vi "BRig_RT__Case_Exp__State_initTrial__v18.vi"(0 "input_dataCurrent":u16[](array[numeric]), 9 "input_dataBlock":u16[][](array[numeric]), 11 "input_dataTrial":u16[][](array[numeric]), 12 "input_dataExp":u16[](array[numeric])) -> (1 "output_iTrial":u16, 2 "output_nTrial":u16, 3 "output_SolenoidReward":bool, 4 "output_dataCurrent":u16[](array[numeric]), 10 "output_dataBlock":u16[][](array[numeric]), 15 "output_dataTrial":u16[][](array[numeric]))   [LabVIEW 2014]
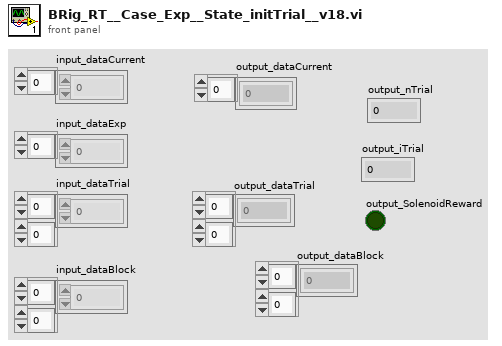
[diagram p1: front panel]
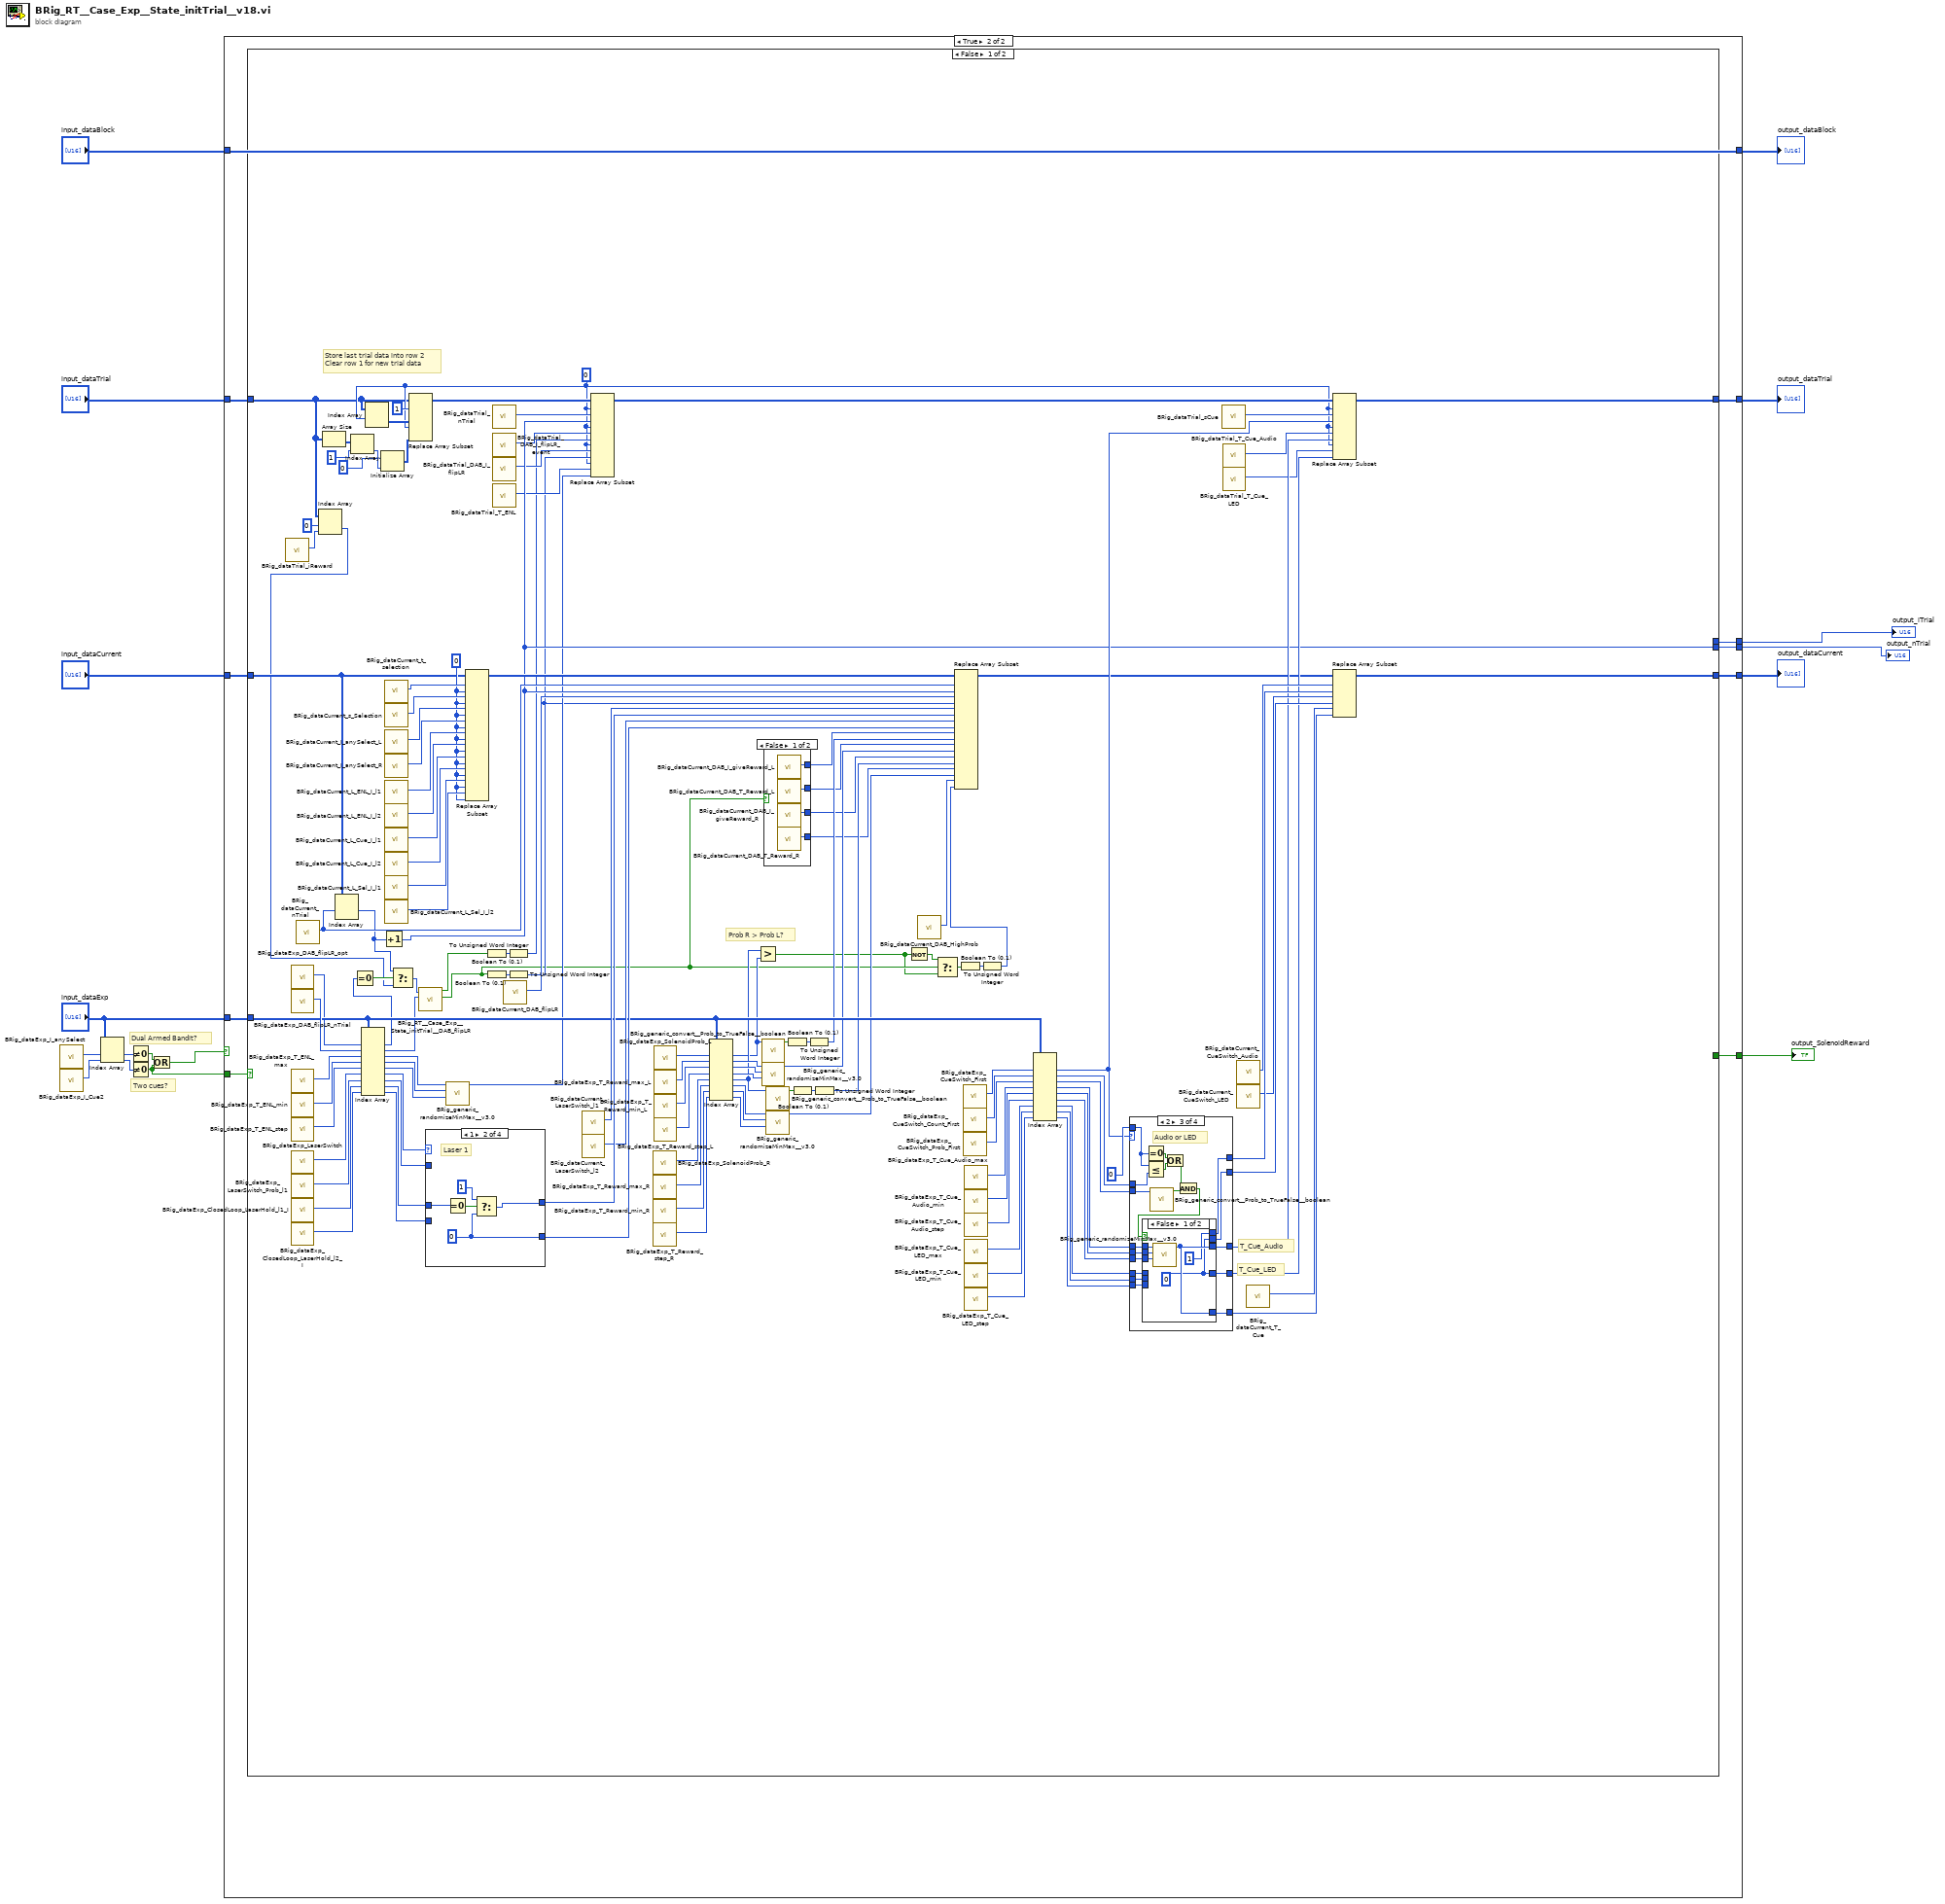
[diagram p0: block diagram]
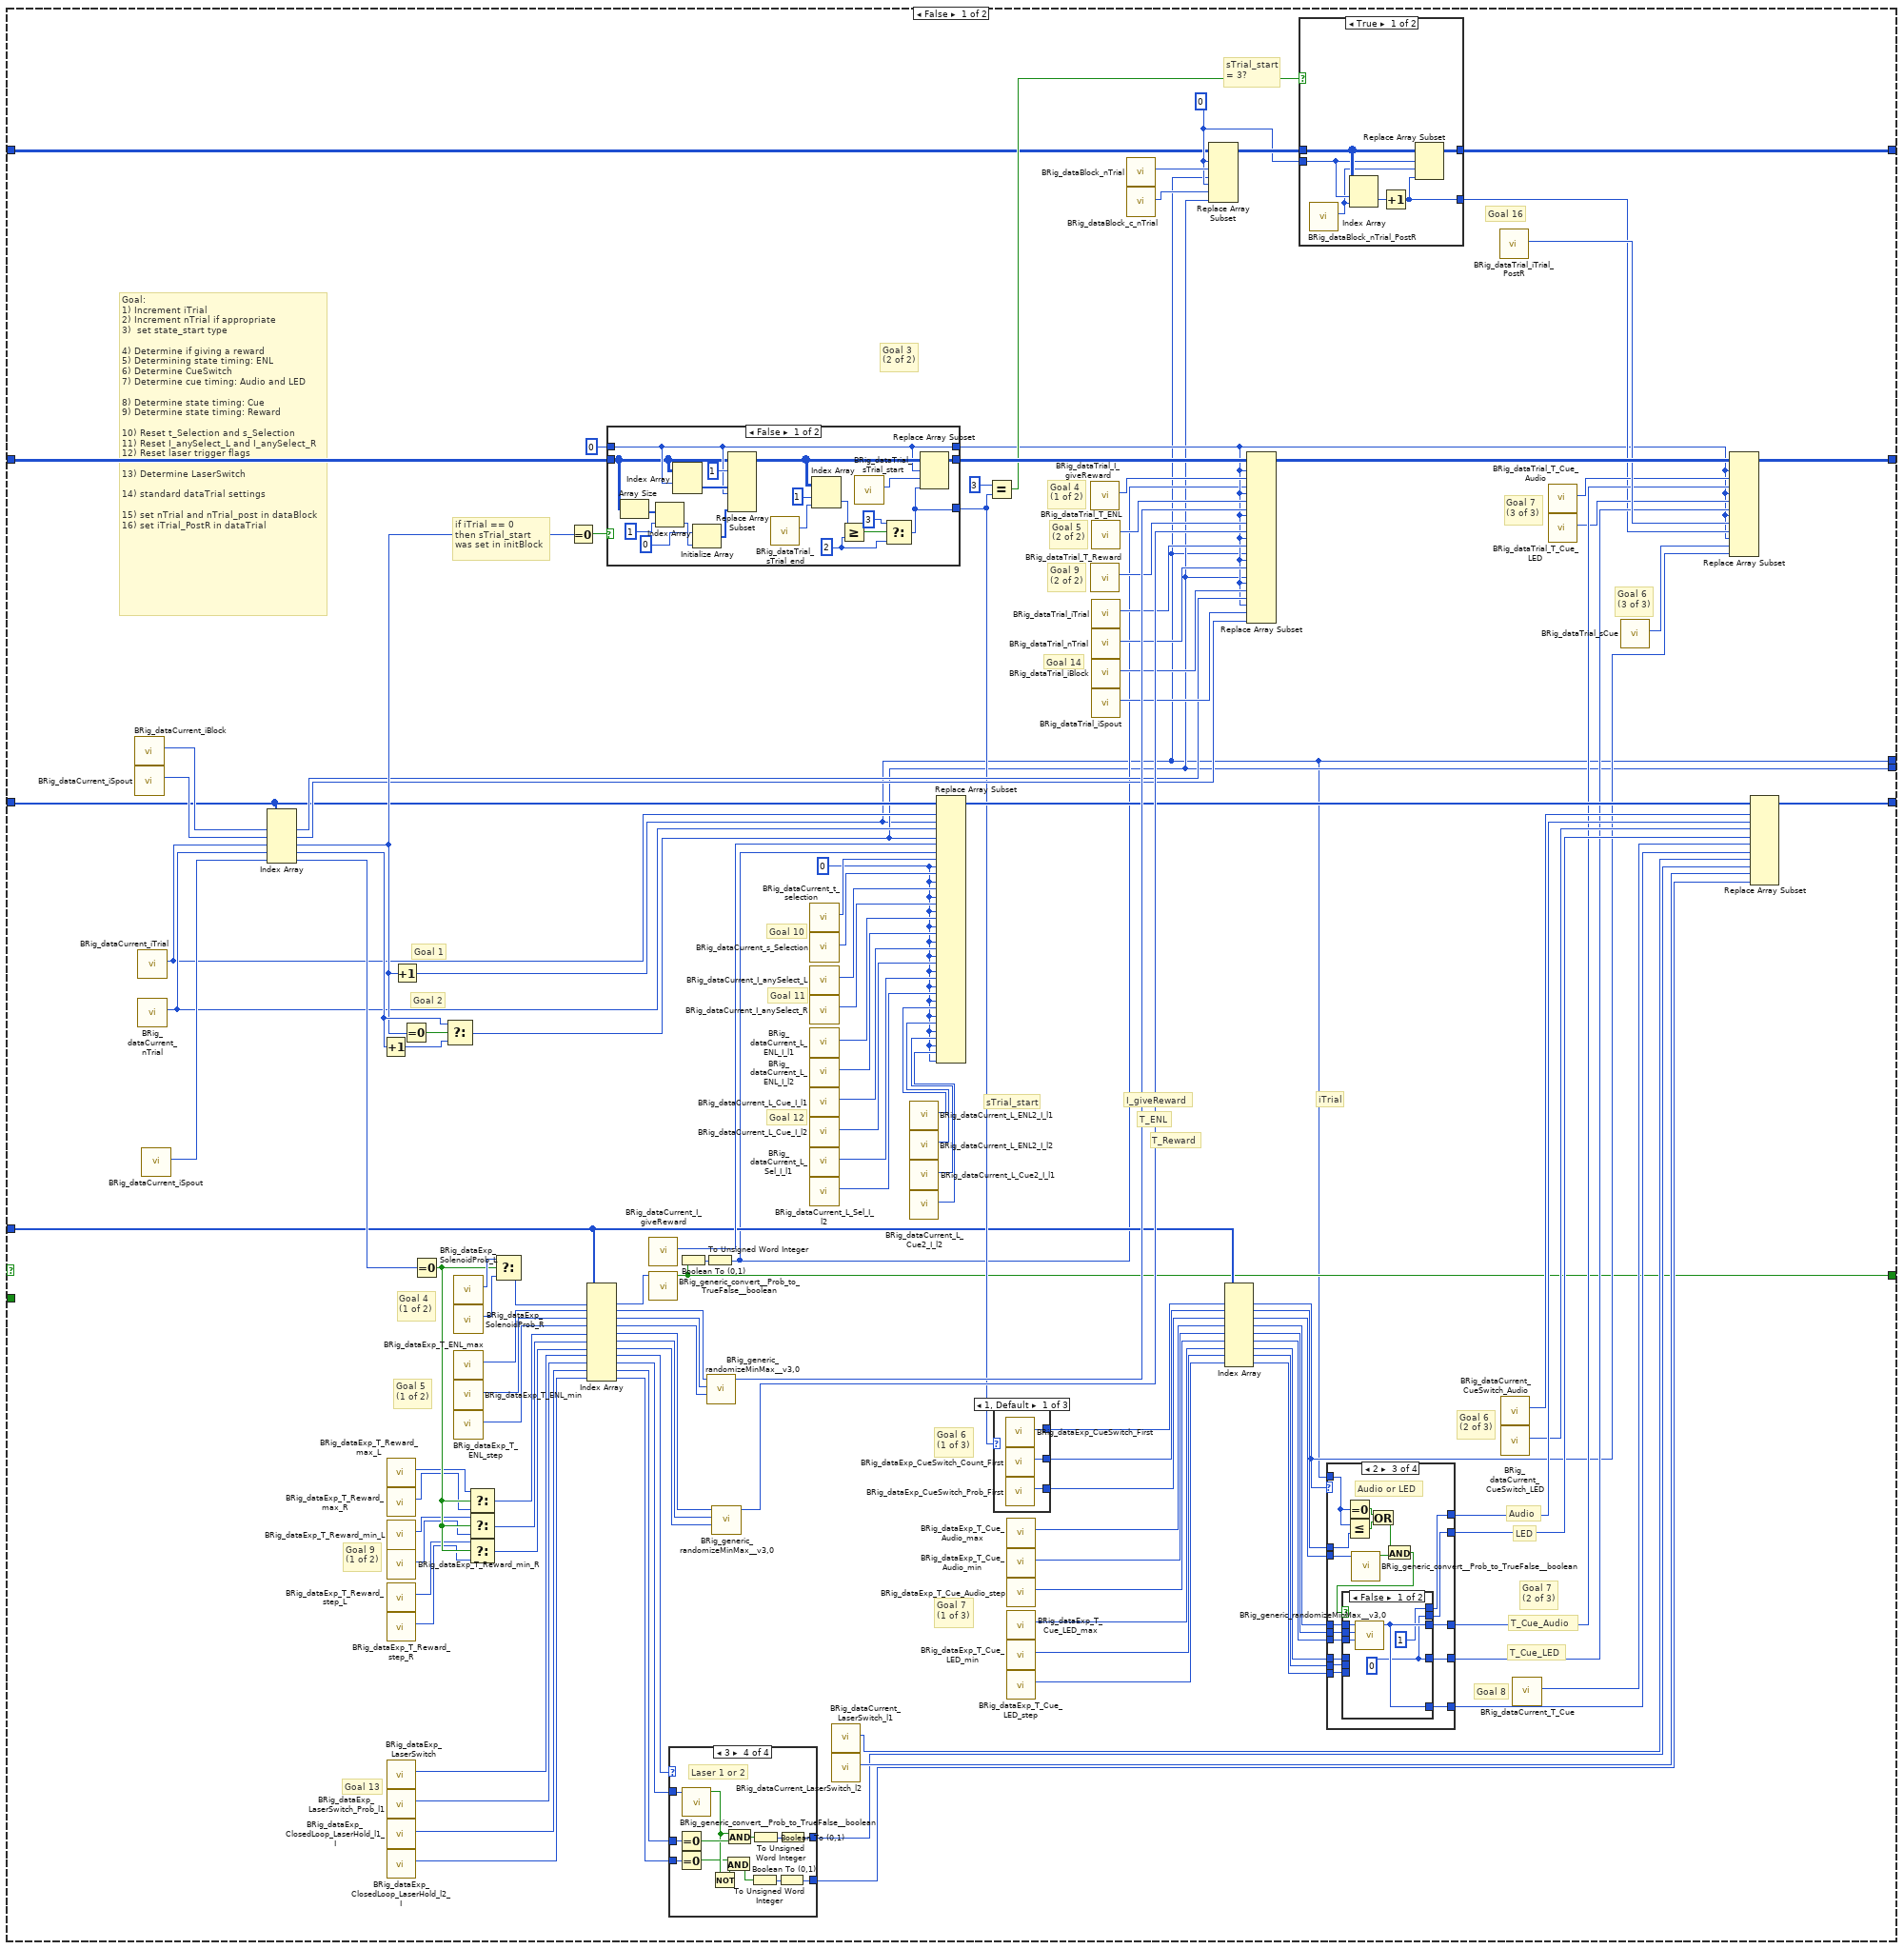
[diagram p2: hidden frame]
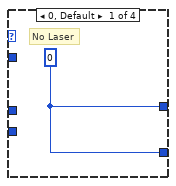
[diagram p4: hidden frame]
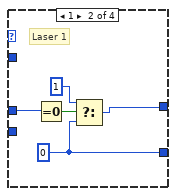
[diagram p5: hidden frame]
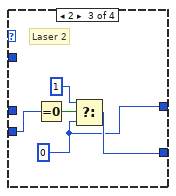
[diagram p6: hidden frame]
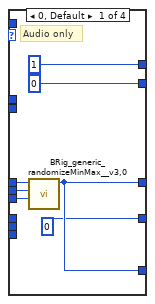
[diagram p7: hidden frame]
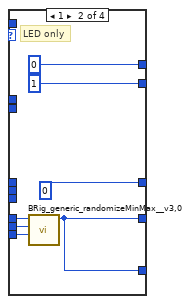
[diagram p8: hidden frame]
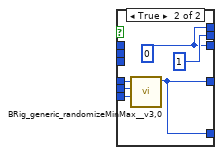
[diagram p9: hidden frame]
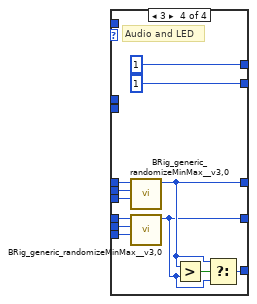
[diagram p10: hidden frame]
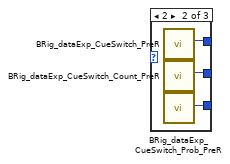
[diagram p11: hidden frame]
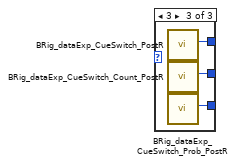
[diagram p12: hidden frame]
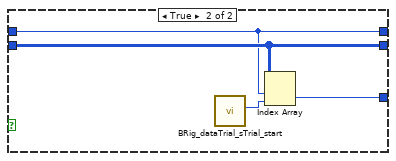
[diagram p13: hidden frame]
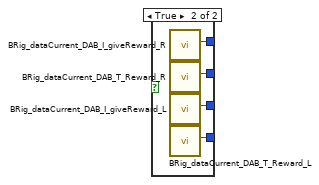
[diagram p14: hidden frame]
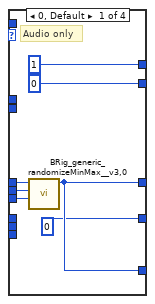
[diagram p15: hidden frame]
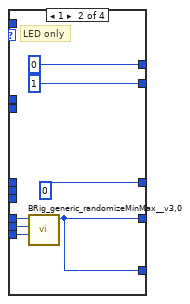
[diagram p16: hidden frame]
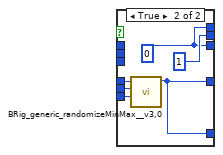
[diagram p17: hidden frame]
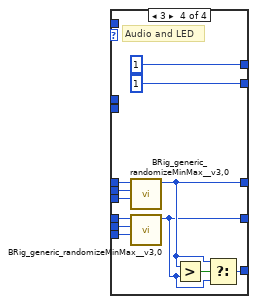
[diagram p18: hidden frame]
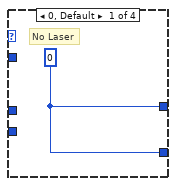
[diagram p19: hidden frame]
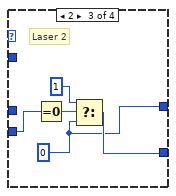
[diagram p20: hidden frame]
diagram:
  # "Two cues?"
  # "Dual Armed Bandit?"
  n1 = call "BRig_dataExp_I_anySelect.vi"() -> ("output_I_anySelect"=w8:i32)  [unwired: 11 in]
  n2 = call "BRig_dataExp_I_Cue2.vi"() -> ("output_I_Cue2"=w6:i32)  [unwired: 11 in]
  n3 = Index Array(array="input_dataExp", index #1=w8, index #2=w6) -> (element #1=w7:u16, element #2=w5:u16)
  n4 = Not Equal To 0?(x=w7) -> (x != 0?=w4:bool)
  n5 = Not Equal To 0?(x=w5) -> (x != 0?=w1:bool)
  n6 = Or(x=w4, y=w1) -> (x .or. y?=w2:bool)
  n7 = case shown="True" w2 {
    tunnel: "input_dataExp" -> [w28 w271]
    tunnel: "input_dataCurrent" -> [w27 w272]
    tunnel: "input_dataTrial" -> [w26 w269]
    tunnel: "input_dataBlock" -> [w25 w275]
    tunnel: [w24 w275] -> w14
    tunnel: [w23 w273] -> w13
    tunnel: [w22 w274] -> w12
    tunnel: [w21 w267] -> w11
    tunnel: [w19 w270] -> w10
    tunnel: [w18 w266] -> w9
    tunnel: w1 -> [_ w268]
    frame False {
      w39 = 0 ("disabled index (row)")
      w31 = u16 0 ("new element/subarray")
      # "Goal 16"
      # "Goal 6\n(3 of 3)"
      # "sTrial_start\n= 3?"
      # "Goal 14"
      # "Goal 13"
      # "iTrial"
      # "Goal 8"
      # "Goal 7\n(3 of 3)"
      # "Goal 7\n(2 of 3)"
      # "Goal 7\n(1 of 3)"
      # "T_Cue_LED"
      # "T_Cue_Audio"
      # "I_giveReward"
      # "Goal 4\n(1 of 2)"
      # "T_Reward"
      # "Goal 9\n(2 of 2)"
      # "Goal 9\n(1 of 2)"
      # "Goal 12"
      # "Goal 11"
      # "Goal 10"
      # "T_ENL"
      # "sTrial_start"
      # "LED"
      # "Audio"
      # "Goal 6\n(2 of 3)"
      # "Goal 6\n(1 of 3)"
      # "Goal 3\n(2 of 2)"
      # "Goal 5\n(2 of 2)"
      # "Goal 5\n(1 of 2)"
      # "Goal 4\n(1 of 2)"
      # "if iTrial == 0\nthen sTrial_start\nwas set in initBlock"
      # "Goal 2"
      # "Goal 1"
      # "Goal:\n1) Increment iTrial\n2) Increment nTrial if appropriate\n3)  set state_start type\n\n4) Determine if giving a reward\n5) Determining state timing: ENL\n6) Determine CueSwitch\n7) Determine cue timing: Audio and LED\n\n8) Determine state timing: Cue\n9) Determine state timing: Reward\n\n10) Reset t_Selection and s_Selection\n11) Reset I_anySelect_L and I_anySelect_R\n12) Reset laser trigger flags\n\n13) Determine LaserSwitch\n\n14) standard dataTrial settings\n\n15) set nTrial and nTrial_post in dataBlock\n16) set iTrial_PostR in dataTrial"
      n8 = call "BRig_dataCurrent_iBlock.vi"() -> ("output_iBlock"=w55:i32)  [unwired: 11 in]
      n9 = call "BRig_dataCurrent_iSpout.vi"() -> ("output_iSpout"=w54:i32)  [unwired: 11 in]
      n10 = call "BRig_dataCurrent_iTrial.vi"() -> ("output_iTrial"=w36:i32)  [unwired: 11 in]
      n11 = call "BRig_dataCurrent_nTrial.vi"() -> ("output_nTrial"=w37:i32)  [unwired: 11 in]
      n12 = call "BRig_dataCurrent_iSpout.vi"() -> ("output_iSpout"=w46:i32)  [unwired: 11 in]
      n13 = Index Array(array=w27, index #1=w55, index #2=w54, index #3=w36, index #4=w37, index #5=w46) -> (element #1=w64:u16, element #2=w63:u16, element #3=w77:u16, element #4=w144:u16, element #5=w45:u16)
      n14 = Increment(x=w144) -> (x+1=w143:u16)
      n15 = call "BRig_dataExp_T_Reward_max_L.vi"() -> ("output_T_Reward_max_L"=w108:i32)  [unwired: 11 in]
      n16 = call "BRig_dataExp_T_Reward_max_R.vi"() -> ("output_T_Reward_max_R"=w107:i32)  [unwired: 11 in]
      n17 = call "BRig_dataExp_T_Reward_min_L.vi"() -> ("output_Tcycle_Reward_min_L"=w106:i32)  [unwired: 11 in]
      n18 = call "BRig_dataExp_T_Reward_min_R.vi"() -> ("output_T_Reward_min_R"=w105:i32)  [unwired: 11 in]
      n19 = call "BRig_dataExp_T_Reward_step_L.vi"() -> ("output_T_Reward_step_L"=w104:i32)  [unwired: 11 in]
      n20 = call "BRig_dataExp_T_Reward_step_R.vi"() -> ("output_T_Reward_step_R"=w103:i32)  [unwired: 11 in]
      n21 = call "BRig_dataExp_LaserSwitch.vi"() -> ("output_LaserSwitch"=w76:i32)  [unwired: 11 in]
      n22 = call "BRig_dataExp_LaserSwitch_Prob_l1.vi"() -> ("output_LaserSwitch_Probability_L1"=w75:i32)  [unwired: 11 in]
      n23 = call "BRig_dataExp_ClosedLoop_LaserHold_l1_I.vi"() -> ("output_CloseLoop_LaserHold_l1_I"=w51:i32)  [unwired: 11 in]
      n24 = call "BRig_dataExp_ClosedLoop_LaserHold_l2_I.vi"() -> ("output_CloseLoop_LaserHold_l2_I"=w50:i32)  [unwired: 11 in]
      n25 = Increment(x=w77) -> (x+1=w18:u16)
      n26 = Equal To 0?(x=w77) -> (x = 0?=w142:bool)
      n27 = Equal To 0?(x=w45) -> (x = 0?=w109:bool)
      n28 = Select(t=w144, s=w142, f=w143) -> (s? t:f=w19:u16)
      n29 = call "BRig_dataExp_SolenoidProb_L.vi"() -> ("output_SolenoidProbability_L"=w139:i32)  [unwired: 11 in]
      n30 = call "BRig_dataExp_SolenoidProb_R.vi"() -> ("output_SolenoidProbability_R"=w138:i32)  [unwired: 11 in]
      n31 = call "BRig_dataExp_T_ENL_max.vi"() -> ("output_T_ENL_max"=w133:i32)  [unwired: 11 in]
      n32 = call "BRig_dataExp_T_ENL_min.vi"() -> ("output_T_ENL_min"=w134:i32)  [unwired: 11 in]
      n33 = call "BRig_dataExp_T_ENL_step.vi"() -> ("output_T_ENL_step"=w135:i32)  [unwired: 11 in]
      n34 = Select(t=w108, s=w109, f=w107) -> (s? t:f=w102:i32)
      n35 = Select(t=w106, s=w109, f=w105) -> (s? t:f=w101:i32)
      n36 = Select(t=w104, s=w109, f=w103) -> (s? t:f=w100:i32)
      n37 = Select(t=w139, s=w109, f=w138) -> (s? t:f=w137:i32)
      n38 = Equal To 0?(x=w77) -> (x = 0?=w141:bool)
      n39 = Index Array(array=w28, index #1=w137, index #2=w133, index #3=w134, index #4=w135, index #5=w102, index #6=w101, index #7=w100, index #8=w76, index #9=w75, index #10=w51, index #11=w50) -> (element #1=w136:u16, element #2=w132:u16, element #3=w131:u16, element #4=w130:u16, element #5=w99:u16, element #6=w98:u16, element #7=w97:u16, element #8=w74:u16, element #9=w73:u16, element #10=w49:u16, element #11=w48:u16)
      n40 = case shown="False" w141 {
        tunnel: w26 -> [w248 w265]
        tunnel: [w259 w265] -> w129
        tunnel: 0 -> [w249 w264]
        tunnel: [w249 w264] -> w29
        tunnel: [w255 w262] -> w30
        frame False {
          w256 = u16 2 ("y")
          n41 = Array Size(array=w248) -> (size(s)=w247:i32[])
          n42 = Index Array(array=w247, index=1) -> (element=w245:i32)
          n43 = Index Array(array=w248, index (row)=w249) -> (element=w252:u16[])  [unwired: 1 in]
          n44 = Initialize Array(u16 0 ("index"), w245) -> (w243:u16[])
          n45 = Replace Array Subset(array=w248, new element #1=w252, index (row) #1=1 ("index (row)"), new element #2=w243, index (row) #2=w249) -> (w250:u16[][])  [unwired: 2 in]
          n46 = call "BRig_dataTrial_sTrial_end.vi"() -> ("output_sTrial_end"=w261:i32)  [unwired: 11 in]
          n47 = Index Array(array=w250, index (row)=1 ("disabled index (row)"), index (col)=w261) -> (element=w260:u16)
          n48 = Greater Or Equal?(x=w260, y=w256) -> (x >= y?=w258:bool)
          n49 = call "BRig_dataTrial_sTrial_start.vi"() -> ("output_sTrial_start"=w254:i32)  [unwired: 11 in]
          n50 = Select(t=u16 3 ("y"), s=w258, f=w256) -> (s? t:f=w255:u16)
          n51 = Replace Array Subset(array=w250, new element=w255, index (row)=w249, index (col)=w254) -> (w259:u16[][])
        }
        frame True {
          n52 = call "BRig_dataTrial_sTrial_start.vi"() -> ("output_sTrial_start"=w263:i32)  [unwired: 11 in]
          n53 = Index Array(array=w265, index (row)=w264, index (col)=w263) -> (element=w262:u16)
        }
      }
      n54 = call "BRig_dataCurrent_I_giveReward.vi"() -> ("output_I_giveReward"=w140:i32)  [unwired: 11 in]
      n55 = call "BRig_generic_convert__Prob_to_TrueFalse__boolean.vi"("input_probability_u16"=w136) -> ("output_TF"=w21:bool)  [unwired: 10 in]
      n56 = case shown="3" w74 {
        tunnel: [w153 w154 w159 w173] -> w71
        tunnel: [w153 w155 w160 w172] -> w70
        tunnel: w73 -> [_ _ _ w176]
        tunnel: w49 -> [_ w158 _ w171]
        tunnel: w48 -> [_ _ w161 w170]
        frame 0, Default {
          w153 = u16 0
          # "No Laser"
        }
        frame 1 {
          w155 = u16 0
          # "Laser 1"
          n57 = Equal To 0?(x=w158) -> (x = 0?=w157:bool)
          n58 = Select(t=u16 1, s=w157, f=w155) -> (s? t:f=w154:u16)
        }
        frame 2 {
          w159 = u16 0
          # "Laser 2"
          n59 = Equal To 0?(x=w161) -> (x = 0?=w163:bool)
          n60 = Select(t=u16 1, s=w163, f=w159) -> (s? t:f=w160:u16)
        }
        frame 3 {
          # "Laser 1 or 2"
          n61 = Equal To 0?(x=w171) -> (x = 0?=w169:bool)
          n62 = Equal To 0?(x=w170) -> (x = 0?=w165:bool)
          n63 = call "BRig_generic_convert__Prob_to_TrueFalse__boolean.vi"("input_probability_u16"=w176) -> ("output_TF"=w168:bool)  [unwired: 10 in]
          n64 = Not(x=w168) -> (.not. x?=w166:bool)
          n65 = And(x=w165, y=w166) -> (x .and. y?=w164:bool)
          n66 = And(x=w168, y=w169) -> (x .and. y?=w167:bool)
          n67 = Boolean To (0,1)(Boolean=w164) -> (0, 1=w175:i16)
          n68 = Boolean To (0,1)(Boolean=w167) -> (0, 1=w174:i16)
          n69 = To Unsigned Word Integer(number=w175) -> (unsigned 16bit integer=w172:u16)
          n70 = To Unsigned Word Integer(number=w174) -> (unsigned 16bit integer=w173:u16)
        }
      }
      n71 = Boolean To (0,1)(Boolean=w21) -> (0, 1=w145:i16)
      n72 = To Unsigned Word Integer(number=w145) -> (unsigned 16bit integer=w20:u16)
      n73 = call "BRig_generic_randomizeMinMax__v3,0.vi"("Input_Increment"=w130, "Input_Min"=w131, "Input_Max"=w132) -> ("Output"=w127:u16)  [unwired: 8 in]
      n74 = call "BRig_generic_randomizeMinMax__v3,0.vi"("Input_Increment"=w97, "Input_Min"=w98, "Input_Max"=w99) -> ("Output"=w95:u16)  [unwired: 8 in]
      n75 = call "BRig_dataCurrent_t_selection.vi"() -> ("output_t_selection"=w119:i32)  [unwired: 11 in]
      n76 = call "BRig_dataCurrent_s_Selection.vi"() -> ("output_s_Selection"=w118:i32)  [unwired: 11 in]
      n77 = call "BRig_dataCurrent_I_anySelect_L.vi"() -> ("output_IanySelect_L"=w117:i32)  [unwired: 11 in]
      n78 = call "BRig_dataCurrent_I_anySelect_R.vi"() -> ("output_IanySelect_R"=w116:i32)  [unwired: 11 in]
      n79 = call "BRig_dataCurrent_L_ENL_I_l1.vi"() -> ("output_L_ENL_I_l1"=w115:i32)  [unwired: 11 in]
      n80 = call "BRig_dataCurrent_L_ENL_I_l2.vi"() -> ("output_L_ENL_I_l2"=w114:i32)  [unwired: 11 in]
      n81 = call "BRig_dataCurrent_L_Cue_I_l1.vi"() -> ("output_L_Cue_I_l1"=w113:i32)  [unwired: 11 in]
      n82 = call "BRig_dataCurrent_L_Cue_I_l2.vi"() -> ("output_L_Cue_I_l2"=w112:i32)  [unwired: 11 in]
      n83 = call "BRig_dataCurrent_L_Sel_I_l1.vi"() -> ("output_L_Sel_I_l1"=w111:i32)  [unwired: 11 in]
      n84 = call "BRig_dataCurrent_L_Sel_I_l2.vi"() -> ("output_L_Sel_I_l2"=w110:i32)  [unwired: 11 in]
      n85 = call "BRig_dataCurrent_LaserSwitch_l1.vi"() -> ("output_LaserSwitch_l1"=w69:i32)  [unwired: 11 in]
      n86 = call "BRig_dataCurrent_LaserSwitch_l2.vi"() -> ("output_LaserSwitch_l2"=w72:i32)  [unwired: 11 in]
      n87 = call "BRig_dataCurrent_L_ENL2_I_l1.vi"() -> ("output_L_ENL2_I_l1"=w35:i32)  [unwired: 11 in]
      n88 = call "BRig_dataCurrent_L_ENL2_I_l2.vi"() -> ("output_L_ENL2_I_l2"=w34:i32)  [unwired: 11 in]
      n89 = call "BRig_dataCurrent_L_Cue2_I_l1.vi"() -> ("output_L_Cue2_I_l1"=w33:i32)  [unwired: 11 in]
      n90 = call "BRig_dataCurrent_L_Cue2_I_l2.vi"() -> ("output_L_Cue2_I_l2"=w32:i32)  [unwired: 11 in]
      n91 = Replace Array Subset(array=w27, new element #1=w18, index #1=w36, new element #2=w19, index #2=w37, new element #3=w20, index #3=w140, new element #4=w31, index #4=w119, new element #5=w31, index #5=w118, new element #6=w31, index #6=w117, new element #7=w31, index #7=w116, new element #8=w31, index #8=w115, new element #9=w31, index #9=w114, new element #10=w31, index #10=w113, new element #11=w31, index #11=w112, new element #12=w31, index #12=w111, new element #13=w31, index #13=w110, new element #14=w31, index #14=w35, new element #15=w31, index #15=w34, new element #16=w31, index #16=w33, new element #17=w31, index #17=w32) -> (w62:u16[])
      n92 = Equal?(x=u16 3 ("y"), y=w30) -> (x = y?=w40:bool)
      n93 = case shown="1, Default" w30 {
        tunnel: [w236 w237 w242] -> w126
        tunnel: [w235 w238 w241] -> w125
        tunnel: [w234 w239 w240] -> w124
        frame 1, Default {
          n94 = call "BRig_dataExp_CueSwitch_First.vi"() -> ("output_CueSwitch_First"=w236:i32)  [unwired: 11 in]
          n95 = call "BRig_dataExp_CueSwitch_Count_First.vi"() -> ("output_CueSwitch_Count_First"=w235:i32)  [unwired: 11 in]
          n96 = call "BRig_dataExp_CueSwitch_Prob_First.vi"() -> ("output_CueSwitch_Prob_First"=w234:i32)  [unwired: 11 in]
        }
        frame 2 {
          n97 = call "BRig_dataExp_CueSwitch_PreR.vi"() -> ("output_CueSwitch_PreR"=w237:i32)  [unwired: 11 in]
          n98 = call "BRig_dataExp_CueSwitch_Count_PreR.vi"() -> ("output_CueSwitch_Count_PreR"=w238:i32)  [unwired: 11 in]
          n99 = call "BRig_dataExp_CueSwitch_Prob_PreR.vi"() -> ("output_CueSwitch_Prob_PreR"=w239:i32)  [unwired: 11 in]
        }
        frame 3 {
          n100 = call "BRig_dataExp_CueSwitch_PostR.vi"() -> ("output_CueSwitch_PostR"=w242:i32)  [unwired: 11 in]
          n101 = call "BRig_dataExp_CueSwitch_Count_PostR.vi"() -> ("output_CueSwitch_Count_PostR"=w241:i32)  [unwired: 11 in]
          n102 = call "BRig_dataExp_CueSwitch_Prob_PostR.vi"() -> ("output_CueSwitch_Prob_PostR"=w240:i32)  [unwired: 11 in]
        }
      }
      n103 = call "BRig_dataExp_T_Cue_Audio_max.vi"() -> ("output_T_Cue_Audio_max"=w93:i32)  [unwired: 11 in]
      n104 = call "BRig_dataExp_T_Cue_Audio_min.vi"() -> ("output_T_Cue_Audio_min"=w92:i32)  [unwired: 11 in]
      n105 = call "BRig_dataExp_T_Cue_Audio_step.vi"() -> ("output_T_Cue_Audio_step"=w91:i32)  [unwired: 11 in]
      n106 = call "BRig_dataExp_T_Cue_LED_max.vi"() -> ("output_T_Cue_LED_max"=w90:i32)  [unwired: 11 in]
      n107 = call "BRig_dataExp_T_Cue_LED_min.vi"() -> ("output_T_Cue_LED_min"=w89:i32)  [unwired: 11 in]
      n108 = call "BRig_dataExp_T_Cue_LED_step.vi"() -> ("output_T_Cue_LED_step"=w88:i32)  [unwired: 11 in]
      n109 = call "BRig_dataTrial_I_giveReward.vi"() -> ("output_I_giveReward"=w94:i32)  [unwired: 11 in]
      n110 = call "BRig_dataTrial_T_Reward.vi"() -> ("output_T_Reward"=w96:i32)  [unwired: 11 in]
      n111 = call "BRig_dataTrial_T_ENL.vi"() -> ("output_T_ENL"=w128:i32)  [unwired: 11 in]
      n112 = call "BRig_dataTrial_iTrial.vi"() -> ("output_iTrial"=w68:i32)  [unwired: 11 in]
      n113 = call "BRig_dataTrial_nTrial.vi"() -> ("output_nTrial"=w67:i32)  [unwired: 11 in]
      n114 = call "BRig_dataTrial_iBlock.vi"() -> ("output_iBlock"=w66:i32)  [unwired: 11 in]
      n115 = call "BRig_dataTrial_iSpout.vi"() -> ("output_iSpout"=w65:i32)  [unwired: 11 in]
      n116 = call "BRig_dataBlock_nTrial.vi"() -> ("output_nTrial"=w42:i32)  [unwired: 11 in]
      n117 = call "BRig_dataBlock_c_nTrial.vi"() -> ("output_c_nTrial"=w41:i32)  [unwired: 11 in]
      n118 = Replace Array Subset(array=w25, new element #1=w18, index (row) #1=w39, index (col) #1=w42, new element #2=w19, index (row) #2=w39, index (col) #2=w41) -> (w43:u16[][])
      n119 = Index Array(array=w28, index #1=w126, index #2=w125, index #3=w124, index #4=w93, index #5=w92, index #6=w91, index #7=w90, index #8=w89, index #9=w88) -> (element #1=w52:u16, element #2=w87:u16, element #3=w86:u16, element #4=w85:u16, element #5=w84:u16, element #6=w83:u16, element #7=w82:u16, element #8=w81:u16, element #9=w80:u16)
      n120 = Replace Array Subset(array=w129, new element #1=w20, index (row) #1=w29, index (col) #1=w94, new element #2=w127, index (row) #2=w29, index (col) #2=w128, new element #3=w95, index (row) #3=w29, index (col) #3=w96, new element #4=w18, index (row) #4=w29, index (col) #4=w68, new element #5=w19, index (row) #5=w29, index (col) #5=w67, new element #6=w64, index (row) #6=w29, index (col) #6=w66, new element #7=w63, index (row) #7=w29, index (col) #7=w65) -> (w61:u16[][])
      n121 = case shown="True" w40 {
        tunnel: w43 -> [w151 w152]
        tunnel: [w149 w152] -> w24
        tunnel: [w146 _] -> w38
        tunnel: w39 -> [w148 _]
        frame True {
          n122 = call "BRig_dataBlock_nTrial_PostR.vi"() -> ("output_nTrial_PostR"=w147:i32)  [unwired: 11 in]
          n123 = Index Array(array=w151, index (row)=w148, index (col)=w147) -> (element=w150:u16)
          n124 = Increment(x=w150) -> (x+1=w146:u16)
          n125 = Replace Array Subset(array=w151, new element=w146, index (row)=w148, index (col)=w147) -> (w149:u16[][])
        }
        frame False {
        }
      }
      n126 = case shown="2" w52 {
        tunnel: [u16 1 u16 0 w195 u16 1] -> w122
        tunnel: [u16 0 u16 1 w194 u16 1] -> w120
        tunnel: w87 -> [_ _ w208 _]
        tunnel: w86 -> [_ _ w205 _]
        tunnel: w85 -> [w181 _ w201 w231]
        tunnel: w84 -> [w180 _ w200 w230]
        tunnel: w83 -> [w179 _ w199 w229]
        tunnel: w82 -> [_ w188 w193 w228]
        tunnel: w81 -> [_ w187 w192 w227]
        tunnel: w80 -> [_ w186 w191 w226]
        tunnel: [w178 u16 0 ("Output") w198 w224] -> w59
        tunnel: [u16 0 ("Output") w185 w196 w223] -> w58
        tunnel: [w178 w185 w197 w222] -> w78
        tunnel: w18 -> [_ _ w209 _]
        frame 0, Default {
          # "Audio only"
          n127 = call "BRig_generic_randomizeMinMax__v3,0.vi"("Input_Increment"=w179, "Input_Min"=w180, "Input_Max"=w181) -> ("Output"=w178:u16)  [unwired: 8 in]
        }
        frame 1 {
          # "LED only"
          n128 = call "BRig_generic_randomizeMinMax__v3,0.vi"("Input_Increment"=w186, "Input_Min"=w187, "Input_Max"=w188) -> ("Output"=w185:u16)  [unwired: 8 in]
        }
        frame 2 {
          # "Audio or LED"
          n129 = Equal To 0?(x=w209) -> (x = 0?=w207:bool)
          n130 = Less Or Equal?(x=w209, y=w208) -> (x <= y?=w206:bool)
          n131 = call "BRig_generic_convert__Prob_to_TrueFalse__boolean.vi"("input_probability_u16"=w205) -> ("output_TF"=w204:bool)  [unwired: 10 in]
          n132 = Or(x=w207, y=w206) -> (x .or. y?=w203:bool)
          n133 = And(x=w203, y=w204) -> (x .and. y?=w202:bool)
          n134 = case shown="False" w202 {
            tunnel: w201 -> [w215 _]
            tunnel: w200 -> [w214 _]
            tunnel: w199 -> [w213 _]
            tunnel: [w212 w216] -> w198
            tunnel: [w212 w218] -> w197
            tunnel: [w210 w218] -> w196
            tunnel: [u16 1 w216] -> w195
            tunnel: [w210 u16 1] -> w194
            tunnel: w193 -> [_ w221]
            tunnel: w192 -> [_ w220]
            tunnel: w191 -> [_ w219]
            frame False {
              w210 = u16 0
              n135 = call "BRig_generic_randomizeMinMax__v3,0.vi"("Input_Increment"=w213, "Input_Min"=w214, "Input_Max"=w215) -> ("Output"=w212:u16)  [unwired: 8 in]
            }
            frame True {
              w216 = u16 0
              n136 = call "BRig_generic_randomizeMinMax__v3,0.vi"("Input_Increment"=w219, "Input_Min"=w220, "Input_Max"=w221) -> ("Output"=w218:u16)  [unwired: 8 in]
            }
          }
        }
        frame 3 {
          # "Audio and LED"
          n137 = call "BRig_generic_randomizeMinMax__v3,0.vi"("Input_Increment"=w229, "Input_Min"=w230, "Input_Max"=w231) -> ("Output"=w224:u16)  [unwired: 8 in]
          n138 = call "BRig_generic_randomizeMinMax__v3,0.vi"("Input_Increment"=w226, "Input_Min"=w227, "Input_Max"=w228) -> ("Output"=w223:u16)  [unwired: 8 in]
          n139 = Greater?(x=w224, y=w223) -> (0:w225:bool)
          n140 = Select(t=w224, s=w225, f=w223) -> (s? t:f=w222:u16)
        }
      }
      n141 = call "BRig_dataTrial_iTrial_PostR.vi"() -> ("output_iTrial_PostR"=w60:i32)  [unwired: 11 in]
      n142 = call "BRig_dataCurrent_CueSwitch_Audio.vi"() -> ("output_CueSwitch_Audio"=w123:i32)  [unwired: 11 in]
      n143 = call "BRig_dataCurrent_CueSwitch_LED.vi"() -> ("output_CueSwitch_LED"=w121:i32)  [unwired: 11 in]
      n144 = call "BRig_dataCurrent_T_Cue.vi"() -> ("output_T_Cue"=w79:i32)  [unwired: 11 in]
      n145 = call "BRig_dataTrial_T_Cue_Audio.vi"() -> ("output_T_Cue_Audio"=w57:i32)  [unwired: 11 in]
      n146 = call "BRig_dataTrial_T_Cue_LED.vi"() -> ("output_T_Cue_LED"=w56:i32)  [unwired: 11 in]
      n147 = call "BRig_dataTrial_sCue.vi"() -> ("output_sCue"=w53:i32)  [unwired: 11 in]
      n148 = Replace Array Subset(array=w61, new element #1=w59, index (row) #1=w29, index (col) #1=w57, new element #2=w58, index (row) #2=w29, index (col) #2=w56, new element #3=w38, index (row) #3=w29, index (col) #3=w60, new element #4=w52, index (row) #4=w29, index (col) #4=w53) -> (w23:u16[][])
      n149 = Replace Array Subset(array=w62, new element #1=w122, index #1=w123, new element #2=w120, index #2=w121, new element #3=w78, index #3=w79, new element #4=w71, index #4=w69, new element #5=w70, index #5=w72) -> (w22:u16[])
    }
    frame True {
      n150 = case shown="False" w268 {
        tunnel: [w364 w512] -> w274
        tunnel: [w363 w511] -> w273
        tunnel: w272 -> [w348 w667]
        tunnel: w271 -> [w339 w544]
        tunnel: [w313 w510] -> w270
        tunnel: w269 -> [w283 w656]
        tunnel: [_ w625] -> w267
        tunnel: [_ w509] -> w266
        frame False {
          w285 = 0
          w391 = u16 0 ("new element/subarray")
          # "Store last trial data into row 2\nClear row 1 for new trial data"
          # "Prob R > Prob L?"
          # "T_Cue_LED"
          # "T_Cue_Audio"
          n151 = call "BRig_dataTrial_iReward.vi"() -> ("output_iReward"=w276:i32)  [unwired: 11 in]
          n152 = call "BRig_dataExp_DAB_flipLR_opt.vi"() -> ("output_DAB_flipLR_opt"=w284:i32)  [unwired: 11 in]
          n153 = call "BRig_dataExp_DAB_flipLR_nTrial.vi"() -> ("output_DAB_flipLR_nTrial"=w344:i32)  [unwired: 11 in]
          n154 = call "BRig_dataExp_T_ENL_max.vi"() -> ("output_T_ENL_max"=w408:i32)  [unwired: 11 in]
          n155 = call "BRig_dataExp_T_ENL_min.vi"() -> ("output_T_ENL_min"=w407:i32)  [unwired: 11 in]
          n156 = call "BRig_dataExp_T_ENL_step.vi"() -> ("output_T_ENL_step"=w406:i32)  [unwired: 11 in]
          n157 = call "BRig_dataExp_LaserSwitch.vi"() -> ("output_LaserSwitch"=w390:i32)  [unwired: 11 in]
          n158 = call "BRig_dataExp_LaserSwitch_Prob_l1.vi"() -> ("output_LaserSwitch_Probability_L1"=w389:i32)  [unwired: 11 in]
          n159 = call "BRig_dataExp_ClosedLoop_LaserHold_l1_I.vi"() -> ("output_CloseLoop_LaserHold_l1_I"=w388:i32)  [unwired: 11 in]
          n160 = call "BRig_dataExp_ClosedLoop_LaserHold_l2_I.vi"() -> ("output_CloseLoop_LaserHold_l2_I"=w387:i32)  [unwired: 11 in]
          n161 = call "BRig_dataCurrent_nTrial.vi"() -> ("output_nTrial"=w346:i32)  [unwired: 11 in]
          n162 = Index Array(array=w283, index (row)=0, index (col)=w276) -> (element=w277:u16)
          n163 = Array Size(array=w283) -> (size(s)=w291:i32[])
          n164 = Index Array(array=w348, index #1=w346) -> (element #1=w279:u16)  [unwired: 1 in, 1 out]
          n165 = Index Array(array=w291, index=1) -> (element=w289:i32)
          n166 = Index Array(array=w339, index #1=w284, index #2=w344, index #3=w408, index #4=w407, index #5=w406, index #6=w390, index #7=w389, index #8=w388, index #9=w387) -> (element #1=w281:u16, element #2=w295:u16, element #3=w404:u16, element #4=w403:u16, element #5=w402:u16, element #6=w386:u16, element #7=w385:u16, element #8=w384:u16, element #9=w383:u16)
          n167 = Equal To 0?(x=w281) -> (x = 0?=w280:bool)
          n168 = Index Array(array=w283, index (row)=w285) -> (element=w293:u16[])  [unwired: 1 in]
          n169 = Initialize Array(u16 0 ("index"), w289) -> (w287:u16[])
          n170 = Increment(x=w279) -> (x+1=w313:u16)
          n171 = call "BRig_dataCurrent_t_selection.vi"() -> ("output_t_selection"=w401:i32)  [unwired: 11 in]
          n172 = call "BRig_dataCurrent_s_Selection.vi"() -> ("output_s_Selection"=w400:i32)  [unwired: 11 in]
          n173 = call "BRig_dataCurrent_I_anySelect_L.vi"() -> ("output_IanySelect_L"=w399:i32)  [unwired: 11 in]
          n174 = call "BRig_dataCurrent_I_anySelect_R.vi"() -> ("output_IanySelect_R"=w398:i32)  [unwired: 11 in]
          n175 = call "BRig_dataCurrent_L_ENL_I_l1.vi"() -> ("output_L_ENL_I_l1"=w397:i32)  [unwired: 11 in]
          n176 = call "BRig_dataCurrent_L_ENL_I_l2.vi"() -> ("output_L_ENL_I_l2"=w396:i32)  [unwired: 11 in]
          n177 = call "BRig_dataCurrent_L_Cue_I_l1.vi"() -> ("output_L_Cue_I_l1"=w395:i32)  [unwired: 11 in]
          n178 = call "BRig_dataCurrent_L_Cue_I_l2.vi"() -> ("output_L_Cue_I_l2"=w394:i32)  [unwired: 11 in]
          n179 = call "BRig_dataCurrent_L_Sel_I_l1.vi"() -> ("output_L_Sel_I_l1"=w393:i32)  [unwired: 11 in]
          n180 = call "BRig_dataCurrent_L_Sel_I_l2.vi"() -> ("output_L_Sel_I_l2"=w392:i32)  [unwired: 11 in]
          n181 = Select(t=w279, s=w280, f=w277) -> (s? t:f=w278:u16)
          n182 = Replace Array Subset(array=w283, new element #1=w293, index (row) #1=1 ("index (row)"), new element #2=w287, index (row) #2=w285) -> (w286:u16[][])  [unwired: 2 in]
          n183 = call "BRig_RT__Case_Exp__State_initTrial__DAB_flipLR.vi"("input_DAB_flipLR_nTrial"=w295, "input_nTrial"=w278) -> ("output_switchedLR"=w301:bool, "output_flipOccurred"=w312:bool)  [unwired: 8 in]
          n184 = case shown="1" w386 {
            tunnel: [w474 w475 w480 w494] -> w342
            tunnel: [w474 w476 w481 w493] -> w340
            tunnel: w385 -> [_ _ _ w497]
            tunnel: w384 -> [_ w479 _ w492]
            tunnel: w383 -> [_ _ w482 w491]
            frame 0, Default {
              w474 = u16 0
              # "No Laser"
            }
            frame 1 {
              w476 = u16 0
              # "Laser 1"
              n185 = Equal To 0?(x=w479) -> (x = 0?=w478:bool)
              n186 = Select(t=u16 1, s=w478, f=w476) -> (s? t:f=w475:u16)
            }
            frame 2 {
              w480 = u16 0
              # "Laser 2"
              n187 = Equal To 0?(x=w482) -> (x = 0?=w484:bool)
              n188 = Select(t=u16 1, s=w484, f=w480) -> (s? t:f=w481:u16)
            }
            frame 3 {
              # "Laser 1 or 2"
              n189 = Equal To 0?(x=w492) -> (x = 0?=w490:bool)
              n190 = Equal To 0?(x=w491) -> (x = 0?=w486:bool)
              n191 = call "BRig_generic_convert__Prob_to_TrueFalse__boolean.vi"("input_probability_u16"=w497) -> ("output_TF"=w489:bool)  [unwired: 10 in]
              n192 = Not(x=w489) -> (.not. x?=w487:bool)
              n193 = And(x=w486, y=w487) -> (x .and. y?=w485:bool)
              n194 = And(x=w489, y=w490) -> (x .and. y?=w488:bool)
              n195 = Boolean To (0,1)(Boolean=w485) -> (0, 1=w496:i16)
              n196 = Boolean To (0,1)(Boolean=w488) -> (0, 1=w495:i16)
              n197 = To Unsigned Word Integer(number=w496) -> (unsigned 16bit integer=w493:u16)
              n198 = To Unsigned Word Integer(number=w495) -> (unsigned 16bit integer=w494:u16)
            }
          }
          n199 = call "BRig_generic_randomizeMinMax__v3,0.vi"("Input_Increment"=w402, "Input_Min"=w403, "Input_Max"=w404) -> ("Output"=w310:u16)  [unwired: 8 in]
          n200 = Replace Array Subset(array=w348, new element #1=w391, index #1=w401, new element #2=w391, index #2=w400, new element #3=w391, index #3=w399, new element #4=w391, index #4=w398, new element #5=w391, index #5=w397, new element #6=w391, index #6=w396, new element #7=w391, index #7=w395, new element #8=w391, index #8=w394, new element #9=w391, index #9=w393, new element #10=w391, index #10=w392) -> ()  [unwired: 1 out]
          n201 = Boolean To (0,1)(Boolean=w312) -> (0, 1=w314:i16)
          n202 = Boolean To (0,1)(Boolean=w301) -> (0, 1=w311:i16)
          n203 = call "BRig_dataTrial_nTrial.vi"() -> ("output_nTrial"=w349:i32)  [unwired: 11 in]
          n204 = call "BRig_dataTrial_DAB_I_flipLR_event.vi"() -> ("output_DAB_I_flipLR_event"=w308:i32)  [unwired: 11 in]
          n205 = call "BRig_dataTrial_DAB_I_flipLR.vi"() -> ("output_DAB_I_flipLR"=w307:i32)  [unwired: 11 in]
          n206 = call "BRig_dataTrial_T_ENL.vi"() -> ("output_T_ENL"=w309:i32)  [unwired: 11 in]
          n207 = call "BRig_dataCurrent_DAB_flipLR.vi"() -> ("output_DAB_flipLR"=w345:i32)  [unwired: 11 in]
          n208 = To Unsigned Word Integer(number=w314) -> (unsigned 16bit integer=w306:u16)
          n209 = To Unsigned Word Integer(number=w311) -> (unsigned 16bit integer=w305:u16)
          n210 = call "BRig_dataCurrent_LaserSwitch_l1.vi"() -> ("output_LaserSwitch_l1"=w343:i32)  [unwired: 11 in]
          n211 = call "BRig_dataCurrent_LaserSwitch_l2.vi"() -> ("output_LaserSwitch_l2"=w341:i32)  [unwired: 11 in]
          n212 = Replace Array Subset(array=w286, new element #1=w313, index (row) #1=w285, index (col) #1=w349, new element #2=w306, index (row) #2=w285, index (col) #2=w308, new element #3=w305, index (row) #3=w285, index (col) #3=w307, new element #4=w310, index (row) #4=w285, index (col) #4=w309) -> (w294:u16[][])
          n213 = call "BRig_dataExp_SolenoidProb_R.vi"() -> ("output_SolenoidProbability_R"=w334:i32)  [unwired: 11 in]
          n214 = call "BRig_dataExp_T_Reward_max_R.vi"() -> ("output_T_Reward_max_R"=w333:i32)  [unwired: 11 in]
          n215 = call "BRig_dataExp_T_Reward_min_R.vi"() -> ("output_T_Reward_min_R"=w332:i32)  [unwired: 11 in]
          n216 = call "BRig_dataExp_T_Reward_step_R.vi"() -> ("output_T_Reward_step_R"=w331:i32)  [unwired: 11 in]
          n217 = call "BRig_dataExp_SolenoidProb_L.vi"() -> ("output_SolenoidProbability_L"=w338:i32)  [unwired: 11 in]
          n218 = call "BRig_dataExp_T_Reward_max_L.vi"() -> ("output_T_Reward_max_L"=w337:i32)  [unwired: 11 in]
          n219 = call "BRig_dataExp_T_Reward_min_L.vi"() -> ("output_Tcycle_Reward_min_L"=w336:i32)  [unwired: 11 in]
          n220 = call "BRig_dataExp_T_Reward_step_L.vi"() -> ("output_T_Reward_step_L"=w335:i32)  [unwired: 11 in]
          n221 = Index Array(array=w339, index #1=w338, index #2=w337, index #3=w336, index #4=w335, index #5=w334, index #6=w333, index #7=w332, index #8=w331) -> (element #1=w303:u16, element #2=w330:u16, element #3=w329:u16, element #4=w328:u16, element #5=w304:u16, element #6=w327:u16, element #7=w326:u16, element #8=w325:u16)
          n222 = Greater?(x=w304, y=w303) -> (0:w300:bool)
          n223 = call "BRig_generic_convert__Prob_to_TrueFalse__boolean.vi"("input_probability_u16"=w303) -> ("output_TF"=w350:bool)  [unwired: 10 in]
          n224 = call "BRig_generic_randomizeMinMax__v3,0.vi"("Input_Increment"=w328, "Input_Min"=w329, "Input_Max"=w330) -> ("Output"=w319:u16)  [unwired: 8 in]
          n225 = case shown="False" w301 {
            tunnel: [w412 w415] -> w322
            tunnel: [w411 w414] -> w320
            tunnel: [w410 w413] -> w318
            tunnel: [w409 w416] -> w316
            frame False {
              n226 = call "BRig_dataCurrent_DAB_I_giveReward_L.vi"() -> ("output_DAB_I_giveReward_L"=w412:i32)  [unwired: 11 in]
              n227 = call "BRig_dataCurrent_DAB_T_Reward_L.vi"() -> ("output_DAB_T_Reward_L"=w411:i32)  [unwired: 11 in]
              n228 = call "BRig_dataCurrent_DAB_I_giveReward_R.vi"() -> ("output_DAB_I_giveReward_R"=w410:i32)  [unwired: 11 in]
              n229 = call "BRig_dataCurrent_DAB_T_Reward_R.vi"() -> ("output_DAB_T_Reward_R"=w409:i32)  [unwired: 11 in]
            }
            frame True {
              n230 = call "BRig_dataCurrent_DAB_I_giveReward_R.vi"() -> ("output_DAB_I_giveReward_R"=w415:i32)  [unwired: 11 in]
              n231 = call "BRig_dataCurrent_DAB_T_Reward_R.vi"() -> ("output_DAB_T_Reward_R"=w414:i32)  [unwired: 11 in]
              n232 = call "BRig_dataCurrent_DAB_I_giveReward_L.vi"() -> ("output_DAB_I_giveReward_L"=w413:i32)  [unwired: 11 in]
              n233 = call "BRig_dataCurrent_DAB_T_Reward_L.vi"() -> ("output_DAB_T_Reward_L"=w416:i32)  [unwired: 11 in]
            }
          }
          n234 = call "BRig_generic_convert__Prob_to_TrueFalse__boolean.vi"("input_probability_u16"=w304) -> ("output_TF"=w323:bool)  [unwired: 10 in]
          n235 = call "BRig_generic_randomizeMinMax__v3,0.vi"("Input_Increment"=w325, "Input_Min"=w326, "Input_Max"=w327) -> ("Output"=w315:u16)  [unwired: 8 in]
          n236 = Boolean To (0,1)(Boolean=w350) -> (0, 1=w405:i16)
          n237 = Boolean To (0,1)(Boolean=w323) -> (0, 1=w324:i16)
          n238 = To Unsigned Word Integer(number=w405) -> (unsigned 16bit integer=w321:u16)
          n239 = To Unsigned Word Integer(number=w324) -> (unsigned 16bit integer=w317:u16)
          n240 = Not(x=w300) -> (.not. x?=w302:bool)
          n241 = call "BRig_dataCurrent_DAB_HighProb.vi"() -> ("output_DAB_HighProb"=w297:i32)  [unwired: 11 in]
          n242 = Select(t=w302, s=w301, f=w300) -> (s? t:f=w298:bool)
          n243 = Boolean To (0,1)(Boolean=w298) -> (0, 1=w299:i16)
          n244 = call "BRig_dataExp_CueSwitch_First.vi"() -> ("output_CueSwitch_First"=w382:i32)  [unwired: 11 in]
          n245 = call "BRig_dataExp_CueSwitch_Count_First.vi"() -> ("output_CueSwitch_Count_First"=w381:i32)  [unwired: 11 in]
          n246 = call "BRig_dataExp_CueSwitch_Prob_First.vi"() -> ("output_CueSwitch_Prob_First"=w380:i32)  [unwired: 11 in]
          n247 = call "BRig_dataExp_T_Cue_Audio_max.vi"() -> ("output_T_Cue_Audio_max"=w379:i32)  [unwired: 11 in]
          n248 = call "BRig_dataExp_T_Cue_Audio_min.vi"() -> ("output_T_Cue_Audio_min"=w378:i32)  [unwired: 11 in]
          n249 = call "BRig_dataExp_T_Cue_Audio_step.vi"() -> ("output_T_Cue_Audio_step"=w377:i32)  [unwired: 11 in]
          n250 = call "BRig_dataExp_T_Cue_LED_max.vi"() -> ("output_T_Cue_LED_max"=w376:i32)  [unwired: 11 in]
          n251 = call "BRig_dataExp_T_Cue_LED_min.vi"() -> ("output_T_Cue_LED_min"=w375:i32)  [unwired: 11 in]
          n252 = call "BRig_dataExp_T_Cue_LED_step.vi"() -> ("output_T_Cue_LED_step"=w374:i32)  [unwired: 11 in]
          n253 = To Unsigned Word Integer(number=w299) -> (unsigned 16bit integer=w296:u16)
          n254 = Replace Array Subset(array=w348, new element #1=w313, index #1=w346, new element #2=w305, index #2=w345, new element #3=w342, index #3=w343, new element #4=w340, index #4=w341, new element #5=w321, index #5=w322, new element #6=w319, index #6=w320, new element #7=w317, index #7=w318, new element #8=w315, index #8=w316, new element #9=w296, index #9=w297) -> (w347:u16[])
          n255 = Index Array(array=w339, index #1=w382, index #2=w381, index #3=w380, index #4=w379, index #5=w378, index #6=w377, index #7=w376, index #8=w375, index #9=w374) -> (element #1=w357:u16, element #2=w372:u16, element #3=w371:u16, element #4=w370:u16, element #5=w369:u16, element #6=w368:u16, element #7=w367:u16, element #8=w366:u16, element #9=w365:u16)
          n256 = case shown="2" w357 {
            tunnel: [u16 1 u16 0 w435 u16 1] -> w361
            tunnel: [u16 0 u16 1 w434 u16 1] -> w359
            tunnel: w372 -> [_ _ w448 _]
            tunnel: w371 -> [_ _ w445 _]
            tunnel: w370 -> [w421 _ w441 w471]
            tunnel: w369 -> [w420 _ w440 w470]
            tunnel: w368 -> [w419 _ w439 w469]
            tunnel: w367 -> [_ w428 w433 w468]
            tunnel: w366 -> [_ w427 w432 w467]
            tunnel: w365 -> [_ w426 w431 w466]
            tunnel: [w418 u16 0 ("Output") w438 w464] -> w355
            tunnel: [u16 0 ("Output") w425 w436 w463] -> w353
            tunnel: [w418 w425 w437 w462] -> w351
            tunnel: u16 0 -> [_ _ w449 _]
            frame 0, Default {
              # "Audio only"
              n257 = call "BRig_generic_randomizeMinMax__v3,0.vi"("Input_Increment"=w419, "Input_Min"=w420, "Input_Max"=w421) -> ("Output"=w418:u16)  [unwired: 8 in]
            }
            frame 1 {
              # "LED only"
              n258 = call "BRig_generic_randomizeMinMax__v3,0.vi"("Input_Increment"=w426, "Input_Min"=w427, "Input_Max"=w428) -> ("Output"=w425:u16)  [unwired: 8 in]
            }
            frame 2 {
              # "Audio or LED"
              n259 = Equal To 0?(x=w449) -> (x = 0?=w447:bool)
              n260 = Less Or Equal?(x=w449, y=w448) -> (x <= y?=w446:bool)
              n261 = call "BRig_generic_convert__Prob_to_TrueFalse__boolean.vi"("input_probability_u16"=w445) -> ("output_TF"=w444:bool)  [unwired: 10 in]
              n262 = Or(x=w447, y=w446) -> (x .or. y?=w443:bool)
              n263 = And(x=w443, y=w444) -> (x .and. y?=w442:bool)
              n264 = case shown="False" w442 {
                tunnel: w441 -> [w455 _]
                tunnel: w440 -> [w454 _]
                tunnel: w439 -> [w453 _]
                tunnel: [w452 w456] -> w438
                tunnel: [w452 w458] -> w437
                tunnel: [w450 w458] -> w436
                tunnel: [u16 1 w456] -> w435
                tunnel: [w450 u16 1] -> w434
                tunnel: w433 -> [_ w461]
                tunnel: w432 -> [_ w460]
                tunnel: w431 -> [_ w459]
                frame False {
                  w450 = u16 0
                  n265 = call "BRig_generic_randomizeMinMax__v3,0.vi"("Input_Increment"=w453, "Input_Min"=w454, "Input_Max"=w455) -> ("Output"=w452:u16)  [unwired: 8 in]
                }
                frame True {
                  w456 = u16 0
                  n266 = call "BRig_generic_randomizeMinMax__v3,0.vi"("Input_Increment"=w459, "Input_Min"=w460, "Input_Max"=w461) -> ("Output"=w458:u16)  [unwired: 8 in]
                }
              }
            }
            frame 3 {
              # "Audio and LED"
              n267 = call "BRig_generic_randomizeMinMax__v3,0.vi"("Input_Increment"=w469, "Input_Min"=w470, "Input_Max"=w471) -> ("Output"=w464:u16)  [unwired: 8 in]
              n268 = call "BRig_generic_randomizeMinMax__v3,0.vi"("Input_Increment"=w466, "Input_Min"=w467, "Input_Max"=w468) -> ("Output"=w463:u16)  [unwired: 8 in]
              n269 = Greater?(x=w464, y=w463) -> (0:w465:bool)
              n270 = Select(t=w464, s=w465, f=w463) -> (s? t:f=w462:u16)
            }
          }
          n271 = call "BRig_dataTrial_sCue.vi"() -> ("output_sCue"=w358:i32)  [unwired: 11 in]
          n272 = call "BRig_dataTrial_T_Cue_Audio.vi"() -> ("output_T_Cue_Audio"=w356:i32)  [unwired: 11 in]
          n273 = call "BRig_dataTrial_T_Cue_LED.vi"() -> ("output_T_Cue_LED"=w354:i32)  [unwired: 11 in]
          n274 = call "BRig_dataCurrent_CueSwitch_Audio.vi"() -> ("output_CueSwitch_Audio"=w362:i32)  [unwired: 11 in]
          n275 = call "BRig_dataCurrent_CueSwitch_LED.vi"() -> ("output_CueSwitch_LED"=w360:i32)  [unwired: 11 in]
          n276 = call "BRig_dataCurrent_T_Cue.vi"() -> ("output_T_Cue"=w352:i32)  [unwired: 11 in]
          n277 = Replace Array Subset(array=w294, new element #1=w357, index (row) #1=w285, index (col) #1=w358, new element #2=w355, index (row) #2=w285, index (col) #2=w356, new element #3=w353, index (row) #3=w285, index (col) #3=w354) -> (w363:u16[][])
          n278 = Replace Array Subset(array=w347, new element #1=w361, index #1=w362, new element #2=w359, index #2=w360, new element #3=w351, index #3=w352) -> (w364:u16[])
        }
        frame True {
          w552 = u16 0 ("index")
          w513 = u16 0 ("new element/subarray")
          w650 = 1 ("index (row)")
          w505 = 0 ("index")
          # "T_Cue_LED"
          # "T_Cue_Audio"
          # "LED"
          # "Audio"
          # "T_Cue_LED"
          # "T_Cue_Audio"
          # "LED"
          # "Audio"
          # "Give Reward?\nL = 1A\nR = 1B"
          # "Time - Reward\nL = 1A\nR = 1B"
          # "Time - ENL2"
          # "Time - ENL1"
          # "Store last trial data into row 2\nClear row 1 for new trial data"
          n279 = call "BRig_dataCurrent_Cue2_I_1A_Sel.vi"() -> ("output_Cue2_I_1A_Sel"=w508:i32)  [unwired: 11 in]
          n280 = call "BRig_dataCurrent_Cue2_I_High_Sel.vi"() -> ("output_Cue2_I_High_Sel"=w507:i32)  [unwired: 11 in]
          n281 = call "BRig_dataCurrent_iTrial.vi"() -> ("output_iTrial"=w664:i32)  [unwired: 11 in]
          n282 = call "BRig_dataCurrent_nTrial.vi"() -> ("output_nTrial"=w585:i32)  [unwired: 11 in]
          n283 = Array Size(array=w656) -> (size(s)=w661:i32[])
          n284 = Index Array(array=w667, index #1=w508, index #2=w507, index #3=w664, index #4=w585) -> (element #1=w503:u16, element #2=w502:u16, element #3=w666:u16, element #4=w665:u16)
          n285 = Index Array(array=w661, index=1) -> (element=w659:i32)
          n286 = Index Array(array=w656, index (row)=w505) -> (element=w663:u16[])  [unwired: 1 in]
          n287 = call "BRig_dataExp_SolenoidProb_L.vi"() -> ("output_SolenoidProbability_L"=w622:i32)  [unwired: 11 in]
          n288 = call "BRig_dataExp_SolenoidProb_R.vi"() -> ("output_SolenoidProbability_R"=w623:i32)  [unwired: 11 in]
          n289 = call "BRig_dataExp_T_ENL_max.vi"() -> ("output_T_ENL_max"=w632:i32)  [unwired: 11 in]
          n290 = call "BRig_dataExp_T_ENL_min.vi"() -> ("output_T_ENL_min"=w631:i32)  [unwired: 11 in]
          n291 = call "BRig_dataExp_T_ENL_step.vi"() -> ("output_T_ENL_step"=w630:i32)  [unwired: 11 in]
          n292 = call "BRig_dataExp_T_ENL2_min.vi"() -> ("output_T_ENL2_min"=w629:i32)  [unwired: 11 in]
          n293 = call "BRig_dataExp_T_ENL2_max.vi"() -> ("output_T_ENL2_max"=w628:i32)  [unwired: 11 in]
          n294 = call "BRig_dataExp_T_ENL2_step.vi"() -> ("output_T_ENL2_step"=w627:i32)  [unwired: 11 in]
          n295 = call "BRig_dataExp_T_Reward_max_L.vi"() -> ("output_T_Reward_max_L"=w614:i32)  [unwired: 11 in]
          n296 = call "BRig_dataExp_T_Reward_max_R.vi"() -> ("output_T_Reward_max_R"=w613:i32)  [unwired: 11 in]
          n297 = call "BRig_dataExp_T_Reward_min_L.vi"() -> ("output_Tcycle_Reward_min_L"=w612:i32)  [unwired: 11 in]
          n298 = call "BRig_dataExp_T_Reward_min_R.vi"() -> ("output_T_Reward_min_R"=w611:i32)  [unwired: 11 in]
          n299 = call "BRig_dataExp_T_Reward_step_L.vi"() -> ("output_T_Reward_step_L"=w610:i32)  [unwired: 11 in]
          n300 = call "BRig_dataExp_T_Reward_step_R.vi"() -> ("output_T_Reward_step_R"=w609:i32)  [unwired: 11 in]
          n301 = call "BRig_dataExp_LaserSwitch.vi"() -> ("output_LaserSwitch"=w602:i32)  [unwired: 11 in]
          n302 = call "BRig_dataExp_LaserSwitch_Prob_l1.vi"() -> ("output_LaserSwitch_Probability_L1"=w601:i32)  [unwired: 11 in]
          n303 = call "BRig_dataExp_ClosedLoop_LaserHold_l1_I.vi"() -> ("output_CloseLoop_LaserHold_l1_I"=w600:i32)  [unwired: 11 in]
          n304 = call "BRig_dataExp_ClosedLoop_LaserHold_l2_I.vi"() -> ("output_CloseLoop_LaserHold_l2_I"=w599:i32)  [unwired: 11 in]
          n305 = Not Equal To 0?(x=w503) -> (x != 0?=w576:bool)
          n306 = Not Equal To 0?(x=w502) -> (x != 0?=w655:bool)
          n307 = Initialize Array(u16 0 ("index"), w659) -> (w657:u16[])
          n308 = Select(t=w622, s=w576, f=w623) -> (s? t:f=w621:i32)
          n309 = Select(t=w614, s=w576, f=w613) -> (s? t:f=w608:i32)
          n310 = Select(t=w612, s=w576, f=w611) -> (s? t:f=w607:i32)
          n311 = Select(t=w610, s=w576, f=w609) -> (s? t:f=w606:i32)
          n312 = Increment(x=w666) -> (x+1=w509:u16)
          n313 = Increment(x=w665) -> (x+1=w510:u16)
          n314 = call "BRig_dataTrial_Cue2_iTrial_1A.vi"() -> ("output_Cue2_iTrial_1A"=w651:i32)  [unwired: 11 in]
          n315 = call "BRig_dataTrial_Cue2_iTrial_1B.vi"() -> ("output_Cue2_iTrial_1B"=w652:i32)  [unwired: 11 in]
          n316 = call "BRig_dataTrial_Cue2_iTrial_High.vi"() -> ("output_Cue2_iTrial_High"=w654:i32)  [unwired: 11 in]
          n317 = call "BRig_dataTrial_Cue2_iTrial_Low.vi"() -> ("output_Cue2_iTrial_Low"=w653:i32)  [unwired: 11 in]
          n318 = Replace Array Subset(array=w656, new element #1=w663, index (row) #1=1 ("index (row)"), new element #2=w657, index (row) #2=w505) -> (w649:u16[][])  [unwired: 2 in]
          n319 = Select(t=w651, s=w576, f=w652) -> (s? t:f=w648:i32)
          n320 = Select(t=w654, s=w655, f=w653) -> (s? t:f=w645:i32)
          n321 = Index Array(array=w544, index #1=w621, index #2=w632, index #3=w631, index #4=w630, index #5=w629, index #6=w628, index #7=w627, index #8=w608, index #9=w607, index #10=w606, index #11=w602, index #12=w601, index #13=w600, index #14=w599) -> (element #1=w624:u16, element #2=w620:u16, element #3=w619:u16, element #4=w618:u16, element #5=w617:u16, element #6=w616:u16, element #7=w615:u16, element #8=w605:u16, element #9=w604:u16, element #10=w603:u16, element #11=w598:u16, element #12=w597:u16, element #13=w596:u16, element #14=w595:u16)
          n322 = Index Array(array=w649, index (row) #1=w650, index (col) #1=w648, index (row) #2=w650, index (col) #2=w645) -> (element #1=w647:u16, element #2=w644:u16)
          n323 = call "BRig_dataTrial_Cue2_I_1A_Sel.vi"() -> ("output_Cue2_I_1A_Sel"=w506:i32)  [unwired: 11 in]
          n324 = call "BRig_dataTrial_Cue2_I_High_Sel.vi"() -> ("output_Cue2_I_High_Sel"=w504:i32)  [unwired: 11 in]
          n325 = Increment(x=w647) -> (x+1=w646:u16)
          n326 = Increment(x=w644) -> (x+1=w643:u16)
          n327 = call "BRig_generic_convert__Prob_to_TrueFalse__boolean.vi"("input_probability_u16"=w624) -> ("output_TF"=w625:bool)  [unwired: 10 in]
          n328 = call "BRig_generic_randomizeMinMax__v3,0.vi"("Input_Increment"=w618, "Input_Min"=w619, "Input_Max"=w620) -> ("Output"=w581:u16)  [unwired: 8 in]
          n329 = call "BRig_generic_randomizeMinMax__v3,0.vi"("Input_Increment"=w615, "Input_Min"=w616, "Input_Max"=w617) -> ("Output"=w579:u16)  [unwired: 8 in]
          n330 = call "BRig_generic_randomizeMinMax__v3,0.vi"("Input_Increment"=w603, "Input_Min"=w604, "Input_Max"=w605) -> ("Output"=w577:u16)  [unwired: 8 in]
          n331 = case shown="3" w598 {
            tunnel: [w782 w783 w788 w802] -> w591
            tunnel: [w782 w784 w789 w801] -> w589
            tunnel: w597 -> [_ _ _ w805]
            tunnel: w596 -> [_ w787 _ w800]
            tunnel: w595 -> [_ _ w790 w799]
            frame 0, Default {
              w782 = u16 0
              # "No Laser"
            }
            frame 1 {
              w784 = u16 0
              # "Laser 1"
              n332 = Equal To 0?(x=w787) -> (x = 0?=w786:bool)
              n333 = Select(t=u16 1, s=w786, f=w784) -> (s? t:f=w783:u16)
            }
            frame 2 {
              w788 = u16 0
              # "Laser 2"
              n334 = Equal To 0?(x=w790) -> (x = 0?=w792:bool)
              n335 = Select(t=u16 1, s=w792, f=w788) -> (s? t:f=w789:u16)
            }
            frame 3 {
              # "Laser 1 or 2"
              n336 = Equal To 0?(x=w800) -> (x = 0?=w798:bool)
              n337 = Equal To 0?(x=w799) -> (x = 0?=w794:bool)
              n338 = call "BRig_generic_convert__Prob_to_TrueFalse__boolean.vi"("input_probability_u16"=w805) -> ("output_TF"=w797:bool)  [unwired: 10 in]
              n339 = Not(x=w797) -> (.not. x?=w795:bool)
              n340 = And(x=w794, y=w795) -> (x .and. y?=w793:bool)
              n341 = And(x=w797, y=w798) -> (x .and. y?=w796:bool)
              n342 = Boolean To (0,1)(Boolean=w793) -> (0, 1=w804:i16)
              n343 = Boolean To (0,1)(Boolean=w796) -> (0, 1=w803:i16)
              n344 = To Unsigned Word Integer(number=w804) -> (unsigned 16bit integer=w801:u16)
              n345 = To Unsigned Word Integer(number=w803) -> (unsigned 16bit integer=w802:u16)
            }
          }
          n346 = Boolean To (0,1)(Boolean=w625) -> (0, 1=w626:i16)
          n347 = Replace Array Subset(array=w667, new element #1=w509, index #1=w664, new element #2=w510, index #2=w585) -> (w594:u16[])
          n348 = Replace Array Subset(array=w649, new element #1=w646, index (row) #1=w505, index (col) #1=w648, new element #2=w643, index (row) #2=w505, index (col) #2=w645, new element #3=w503, index (row) #3=w505, index (col) #3=w506, new element #4=w502, index (row) #4=w505, index (col) #4=w504) -> (w588:u16[][])
          n349 = To Unsigned Word Integer(number=w626) -> (unsigned 16bit integer=w583:u16)
          n350 = call "BRig_dataTrial_iTrial.vi"() -> ("output_iTrial"=w587:i32)  [unwired: 11 in]
          n351 = call "BRig_dataTrial_nTrial.vi"() -> ("output_nTrial"=w586:i32)  [unwired: 11 in]
          n352 = call "BRig_dataTrial_I_giveReward.vi"() -> ("output_I_giveReward"=w584:i32)  [unwired: 11 in]
          n353 = call "BRig_dataTrial_T_ENL.vi"() -> ("output_T_ENL"=w582:i32)  [unwired: 11 in]
          n354 = call "BRig_dataTrial_T_ENL2.vi"() -> ("output_T_ENL2"=w580:i32)  [unwired: 11 in]
          n355 = call "BRig_dataTrial_T_Reward.vi"() -> ("output_T_Reward"=w578:i32)  [unwired: 11 in]
          n356 = call "BRig_dataCurrent_LaserSwitch_l1.vi"() -> ("output_LaserSwitch_l1"=w592:i32)  [unwired: 11 in]
          n357 = call "BRig_dataCurrent_LaserSwitch_l2.vi"() -> ("output_LaserSwitch_l2"=w590:i32)  [unwired: 11 in]
          n358 = Replace Array Subset(array=w588, new element #1=w509, index (row) #1=w505, index (col) #1=w587, new element #2=w510, index (row) #2=w505, index (col) #2=w586, new element #3=w583, index (row) #3=w505, index (col) #3=w584, new element #4=w581, index (row) #4=w505, index (col) #4=w582, new element #5=w579, index (row) #5=w505, index (col) #5=w580, new element #6=w577, index (row) #6=w505, index (col) #6=w578) -> (w530:u16[][])
          n359 = Replace Array Subset(array=w594, new element #1=w591, index #1=w592, new element #2=w589, index #2=w590) -> (w593:u16[])
          n360 = call "BRig_dataExp_CueSwitch_First.vi"() -> ("output_CueSwitch_First"=w575:i32)  [unwired: 11 in]
          n361 = call "BRig_dataExp_CueSwitch_PreR.vi"() -> ("output_CueSwitch_PreR"=w501:i32)  [unwired: 11 in]
          n362 = call "BRig_dataExp_CueSwitch_Prob_First.vi"() -> ("output_CueSwitch_Prob_First"=w574:i32)  [unwired: 11 in]
          n363 = call "BRig_dataExp_CueSwitch_Prob_PreR.vi"() -> ("output_CueSwitch_Prob_PreR"=w500:i32)  [unwired: 11 in]
          n364 = call "BRig_dataExp_T_Cue_Audio_max.vi"() -> ("output_T_Cue_Audio_max"=w571:i32)  [unwired: 11 in]
          n365 = call "BRig_dataExp_T_Cue_Audio_min.vi"() -> ("output_T_Cue_Audio_min"=w570:i32)  [unwired: 11 in]
          n366 = call "BRig_dataExp_T_Cue_Audio_step.vi"() -> ("output_T_Cue_Audio_step"=w569:i32)  [unwired: 11 in]
          n367 = call "BRig_dataExp_T_Cue_LED_max.vi"() -> ("output_T_Cue_LED_max"=w568:i32)  [unwired: 11 in]
          n368 = call "BRig_dataExp_T_Cue_LED_min.vi"() -> ("output_T_Cue_LED_min"=w567:i32)  [unwired: 11 in]
          n369 = call "BRig_dataExp_T_Cue_LED_step.vi"() -> ("output_T_Cue_LED_step"=w566:i32)  [unwired: 11 in]
          n370 = call "BRig_dataExp_CueSwitch_PostR.vi"() -> ("output_CueSwitch_PostR"=w499:i32)  [unwired: 11 in]
          n371 = call "BRig_dataExp_CueSwitch_Prob_PostR.vi"() -> ("output_CueSwitch_Prob_PostR"=w498:i32)  [unwired: 11 in]
          n372 = call "BRig_dataExp_T_Cue2_Audio_max.vi"() -> ("output_T_Cue2_Audio_max"=w558:i32)  [unwired: 11 in]
          n373 = call "BRig_dataExp_T_Cue2_Audio_min.vi"() -> ("output_T_Cue2_Audio_min"=w557:i32)  [unwired: 11 in]
          n374 = call "BRig_dataExp_T_Cue2_Audio_step.vi"() -> ("output_T_Cue2_Audio_step"=w556:i32)  [unwired: 11 in]
          n375 = call "BRig_dataExp_T_Cue2_LED_max.vi"() -> ("output_T_Cue2_LED_max"=w555:i32)  [unwired: 11 in]
          n376 = call "BRig_dataExp_T_Cue2_LED_min.vi"() -> ("output_T_Cue2_LED_min"=w554:i32)  [unwired: 11 in]
          n377 = call "BRig_dataExp_T_Cue2_LED_step.vi"() -> ("output_T_Cue2_LED_step"=w553:i32)  [unwired: 11 in]
          n378 = Select(t=w575, s=w576, f=w501) -> (s? t:f=w573:i32)
          n379 = Select(t=w574, s=w576, f=w500) -> (s? t:f=w572:i32)
          n380 = call "BRig_dataCurrent_t_selection.vi"() -> ("output_t_selection"=w642:i32)  [unwired: 11 in]
          n381 = call "BRig_dataCurrent_s_Selection.vi"() -> ("output_s_Selection"=w641:i32)  [unwired: 11 in]
          n382 = call "BRig_dataCurrent_I_anySelect_L.vi"() -> ("output_IanySelect_L"=w640:i32)  [unwired: 11 in]
          n383 = call "BRig_dataCurrent_I_anySelect_R.vi"() -> ("output_IanySelect_R"=w639:i32)  [unwired: 11 in]
          n384 = call "BRig_dataCurrent_L_ENL_I_l1.vi"() -> ("output_L_ENL_I_l1"=w638:i32)  [unwired: 11 in]
          n385 = call "BRig_dataCurrent_L_ENL_I_l2.vi"() -> ("output_L_ENL_I_l2"=w637:i32)  [unwired: 11 in]
          n386 = call "BRig_dataCurrent_L_Cue_I_l1.vi"() -> ("output_L_Cue_I_l1"=w636:i32)  [unwired: 11 in]
          n387 = call "BRig_dataCurrent_L_Cue_I_l2.vi"() -> ("output_L_Cue_I_l2"=w635:i32)  [unwired: 11 in]
          n388 = call "BRig_dataCurrent_L_Sel_I_l1.vi"() -> ("output_L_Sel_I_l1"=w634:i32)  [unwired: 11 in]
          n389 = call "BRig_dataCurrent_L_Sel_I_l2.vi"() -> ("output_L_Sel_I_l2"=w633:i32)  [unwired: 11 in]
          n390 = Index Array(array=w544, index #1=w573, index #2=w572, index #3=w571, index #4=w570, index #5=w569, index #6=w568, index #7=w567, index #8=w566, index #9=w499, index #10=w498, index #11=w558, index #12=w557, index #13=w556, index #14=w555, index #15=w554, index #16=w553) -> (element #1=w529:u16, element #2=w565:u16, element #3=w564:u16, element #4=w563:u16, element #5=w562:u16, element #6=w561:u16, element #7=w560:u16, element #8=w559:u16, element #9=w523:u16, element #10=w551:u16, element #11=w550:u16, element #12=w549:u16, element #13=w548:u16, element #14=w547:u16, element #15=w546:u16, element #16=w545:u16)
          n391 = call "BRig_dataCurrent_L_ENL2_I_l1.vi"() -> ("output_L_ENL2_I_l1"=w517:i32)  [unwired: 11 in]
          n392 = call "BRig_dataCurrent_L_ENL2_I_l2.vi"() -> ("output_L_ENL2_I_l2"=w516:i32)  [unwired: 11 in]
          n393 = call "BRig_dataCurrent_L_Cue2_I_l1.vi"() -> ("output_L_Cue2_I_l1"=w515:i32)  [unwired: 11 in]
          n394 = call "BRig_dataCurrent_L_Cue2_I_l2.vi"() -> ("output_L_Cue2_I_l2"=w514:i32)  [unwired: 11 in]
          n395 = Replace Array Subset(array=w593, new element #1=w513, index #1=w642, new element #2=w513, index #2=w641, new element #3=w513, index #3=w640, new element #4=w513, index #4=w639, new element #5=w513, index #5=w638, new element #6=w513, index #6=w637, new element #7=w513, index #7=w636, new element #8=w513, index #8=w635, new element #9=w513, index #9=w634, new element #10=w513, index #10=w633, new element #11=w513, index #11=w517, new element #12=w513, index #12=w516, new element #13=w513, index #13=w515, new element #14=w513, index #14=w514) -> (w531:u16[])
          n396 = case shown="2" w529 {
            tunnel: [u16 1 u16 0 w743 u16 1] -> w542
            tunnel: [u16 0 u16 1 w742 u16 1] -> w540
            tunnel: w552 -> [_ _ w756 _]
            tunnel: w565 -> [_ _ w753 _]
            tunnel: w564 -> [w729 _ w749 w779]
            tunnel: w563 -> [w728 _ w748 w778]
            tunnel: w562 -> [w727 _ w747 w777]
            tunnel: w561 -> [_ w736 w741 w776]
            tunnel: w560 -> [_ w735 w740 w775]
            tunnel: w559 -> [_ w734 w739 w774]
            tunnel: [w726 u16 0 ("Output") w746 w772] -> w526
            tunnel: [u16 0 ("Output") w733 w744 w771] -> w524
            tunnel: [w726 w733 w745 w770] -> w538
            tunnel: w552 -> [_ _ w757 _]
            frame 0, Default {
              # "Audio only"
              n397 = call "BRig_generic_randomizeMinMax__v3,0.vi"("Input_Increment"=w727, "Input_Min"=w728, "Input_Max"=w729) -> ("Output"=w726:u16)  [unwired: 8 in]
            }
            frame 1 {
              # "LED only"
              n398 = call "BRig_generic_randomizeMinMax__v3,0.vi"("Input_Increment"=w734, "Input_Min"=w735, "Input_Max"=w736) -> ("Output"=w733:u16)  [unwired: 8 in]
            }
            frame 2 {
              # "Audio or LED"
              n399 = Equal To 0?(x=w757) -> (x = 0?=w755:bool)
              n400 = Less Or Equal?(x=w757, y=w756) -> (x <= y?=w754:bool)
              n401 = call "BRig_generic_convert__Prob_to_TrueFalse__boolean.vi"("input_probability_u16"=w753) -> ("output_TF"=w752:bool)  [unwired: 10 in]
              n402 = Or(x=w755, y=w754) -> (x .or. y?=w751:bool)
              n403 = And(x=w751, y=w752) -> (x .and. y?=w750:bool)
              n404 = case shown="False" w750 {
                tunnel: w749 -> [w763 _]
                tunnel: w748 -> [w762 _]
                tunnel: w747 -> [w761 _]
                tunnel: [w760 w764] -> w746
                tunnel: [w760 w766] -> w745
                tunnel: [w758 w766] -> w744
                tunnel: [u16 1 w764] -> w743
                tunnel: [w758 u16 1] -> w742
                tunnel: w741 -> [_ w769]
                tunnel: w740 -> [_ w768]
                tunnel: w739 -> [_ w767]
                frame False {
                  w758 = u16 0
                  n405 = call "BRig_generic_randomizeMinMax__v3,0.vi"("Input_Increment"=w761, "Input_Min"=w762, "Input_Max"=w763) -> ("Output"=w760:u16)  [unwired: 8 in]
                }
                frame True {
                  w764 = u16 0
                  n406 = call "BRig_generic_randomizeMinMax__v3,0.vi"("Input_Increment"=w767, "Input_Min"=w768, "Input_Max"=w769) -> ("Output"=w766:u16)  [unwired: 8 in]
                }
              }
            }
            frame 3 {
              # "Audio and LED"
              n407 = call "BRig_generic_randomizeMinMax__v3,0.vi"("Input_Increment"=w777, "Input_Min"=w778, "Input_Max"=w779) -> ("Output"=w772:u16)  [unwired: 8 in]
              n408 = call "BRig_generic_randomizeMinMax__v3,0.vi"("Input_Increment"=w774, "Input_Min"=w775, "Input_Max"=w776) -> ("Output"=w771:u16)  [unwired: 8 in]
              n409 = Greater?(x=w772, y=w771) -> (0:w773:bool)
              n410 = Select(t=w772, s=w773, f=w771) -> (s? t:f=w770:u16)
            }
          }
          n411 = case shown="2" w523 {
            tunnel: [u16 1 u16 0 w686 u16 1] -> w536
            tunnel: [u16 0 u16 1 w685 u16 1] -> w534
            tunnel: w552 -> [_ _ w699 _]
            tunnel: w551 -> [_ _ w696 _]
            tunnel: w550 -> [w672 _ w692 w722]
            tunnel: w549 -> [w671 _ w691 w721]
            tunnel: w548 -> [w670 _ w690 w720]
            tunnel: w547 -> [_ w679 w684 w719]
            tunnel: w546 -> [_ w678 w683 w718]
            tunnel: w545 -> [_ w677 w682 w717]
            tunnel: [w669 u16 0 ("Output") w689 w715] -> w520
            tunnel: [u16 0 ("Output") w676 w687 w714] -> w518
            tunnel: [w669 w676 w688 w713] -> w532
            tunnel: w552 -> [_ _ w700 _]
            frame 0, Default {
              # "Audio only"
              n412 = call "BRig_generic_randomizeMinMax__v3,0.vi"("Input_Increment"=w670, "Input_Min"=w671, "Input_Max"=w672) -> ("Output"=w669:u16)  [unwired: 8 in]
            }
            frame 1 {
              # "LED only"
              n413 = call "BRig_generic_randomizeMinMax__v3,0.vi"("Input_Increment"=w677, "Input_Min"=w678, "Input_Max"=w679) -> ("Output"=w676:u16)  [unwired: 8 in]
            }
            frame 2 {
              # "Audio or LED"
              n414 = Equal To 0?(x=w700) -> (x = 0?=w698:bool)
              n415 = Less Or Equal?(x=w700, y=w699) -> (x <= y?=w697:bool)
              n416 = call "BRig_generic_convert__Prob_to_TrueFalse__boolean.vi"("input_probability_u16"=w696) -> ("output_TF"=w695:bool)  [unwired: 10 in]
              n417 = Or(x=w698, y=w697) -> (x .or. y?=w694:bool)
              n418 = And(x=w694, y=w695) -> (x .and. y?=w693:bool)
              n419 = case shown="False" w693 {
                tunnel: w692 -> [w706 _]
                tunnel: w691 -> [w705 _]
                tunnel: w690 -> [w704 _]
                tunnel: [w703 w707] -> w689
                tunnel: [w703 w709] -> w688
                tunnel: [w701 w709] -> w687
                tunnel: [u16 1 w707] -> w686
                tunnel: [w701 u16 1] -> w685
                tunnel: w684 -> [_ w712]
                tunnel: w683 -> [_ w711]
                tunnel: w682 -> [_ w710]
                frame False {
                  w701 = u16 0
                  n420 = call "BRig_generic_randomizeMinMax__v3,0.vi"("Input_Increment"=w704, "Input_Min"=w705, "Input_Max"=w706) -> ("Output"=w703:u16)  [unwired: 8 in]
                }
                frame True {
                  w707 = u16 0
                  n421 = call "BRig_generic_randomizeMinMax__v3,0.vi"("Input_Increment"=w710, "Input_Min"=w711, "Input_Max"=w712) -> ("Output"=w709:u16)  [unwired: 8 in]
                }
              }
            }
            frame 3 {
              # "Audio and LED"
              n422 = call "BRig_generic_randomizeMinMax__v3,0.vi"("Input_Increment"=w720, "Input_Min"=w721, "Input_Max"=w722) -> ("Output"=w715:u16)  [unwired: 8 in]
              n423 = call "BRig_generic_randomizeMinMax__v3,0.vi"("Input_Increment"=w717, "Input_Min"=w718, "Input_Max"=w719) -> ("Output"=w714:u16)  [unwired: 8 in]
              n424 = Greater?(x=w715, y=w714) -> (0:w716:bool)
              n425 = Select(t=w715, s=w716, f=w714) -> (s? t:f=w713:u16)
            }
          }
          n426 = call "BRig_dataTrial_sCue.vi"() -> ("output_sCue"=w528:i32)  [unwired: 11 in]
          n427 = call "BRig_dataCurrent_CueSwitch_Audio.vi"() -> ("output_CueSwitch_Audio"=w543:i32)  [unwired: 11 in]
          n428 = call "BRig_dataCurrent_CueSwitch_LED.vi"() -> ("output_CueSwitch_LED"=w541:i32)  [unwired: 11 in]
          n429 = call "BRig_dataTrial_T_Cue_Audio.vi"() -> ("output_T_Cue_Audio"=w527:i32)  [unwired: 11 in]
          n430 = call "BRig_dataTrial_T_Cue_LED.vi"() -> ("output_T_Cue_LED"=w525:i32)  [unwired: 11 in]
          n431 = call "BRig_dataCurrent_T_Cue.vi"() -> ("output_T_Cue"=w539:i32)  [unwired: 11 in]
          n432 = call "BRig_dataTrial_sCue2.vi"() -> ("output_sCue2"=w522:i32)  [unwired: 11 in]
          n433 = call "BRig_dataCurrent_Cue2Switch_Audio.vi"() -> ("output_Cue2Switch_Audio"=w537:i32)  [unwired: 11 in]
          n434 = call "BRig_dataCurrent_Cue2Switch_LED.vi"() -> ("output_Cue2Switch_LED"=w535:i32)  [unwired: 11 in]
          n435 = call "BRig_dataTrial_T_Cue2_Audio.vi"() -> ("output_T_Cue2_Audio"=w521:i32)  [unwired: 11 in]
          n436 = call "BRig_dataTrial_T_Cue2_LED.vi"() -> ("output_T_Cue2_LED"=w519:i32)  [unwired: 11 in]
          n437 = call "BRig_dataCurrent_T_Cue2.vi"() -> ("output_T_Cue2"=w533:i32)  [unwired: 11 in]
          n438 = Replace Array Subset(array=w531, new element #1=w542, index #1=w543, new element #2=w540, index #2=w541, new element #3=w538, index #3=w539, new element #4=w536, index #4=w537, new element #5=w534, index #5=w535, new element #6=w532, index #6=w533) -> (w512:u16[])
          n439 = Replace Array Subset(array=w530, new element #1=w529, index (row) #1=w505, index (col) #1=w528, new element #2=w526, index (row) #2=w505, index (col) #2=w527, new element #3=w524, index (row) #3=w505, index (col) #3=w525, new element #4=w523, index (row) #4=w505, index (col) #4=w522, new element #5=w520, index (row) #5=w505, index (col) #5=w521, new element #6=w518, index (row) #6=w505, index (col) #6=w519) -> (w511:u16[][])
        }
      }
    }
  }
  "output_dataBlock" <- w14
  "output_dataTrial" <- w13
  "output_dataCurrent" <- w12
  "output_SolenoidReward" <- w11
  "output_nTrial" <- w10
  "output_iTrial" <- w9
